vi "Automated5.vi"() -> ()   [LabVIEW 2018]
uses:
  <vilib>/Platform/TimedLoop/XDataNode/timing_clust.ctl
  <vilib>/Platform/TimedLoop/XDataNode/nitl_modes.ctl
  <vilib>/Platform/TimedLoop/XDataNode/wakeup.ctl
  <vilib>/DAQmx/read.llb/DAQmx Read (Analog 1D DBL NChan 1Samp).vi
  <vilib>/DAQmx/create/channels.llb/DAQmx Create Channel (AI-Voltage-Basic).vi
  <vilib>/Enthought/Python Integration Toolkit/api/Unpack Double.vi
  <vilib>/DAQmx/miscellaneous.llb/DAQmx Fill In Error Info.vi
  <vilib>/platform/TimedLoop/XDataNode/XDataNode.xnode
  Program Files/National Instruments/LabVIEW 2015/instr.lib/Omega CN7500/Omega CN7500.lvlib
  <instrlib>/Brooks DLL 64bit/0254 64bit/BrooksDLL64.dll
  <vilib>/Platform/TimedLoop/XDataNode/XDNodeRunTimeDep.lvlib
  <vilib>/Enthought/Python Integration Toolkit/Python Integration Toolkit.lvlib
panel:
  out "CH4/He Set Flow 9":dbl
  out "N2 Set Flow 9":dbl
  out "CH4/He Set Flow 8":dbl
  out "N2 Set Flow 8":dbl
  out "CH4/He Set Flow 7":dbl
  out "N2 Set Flow 7":dbl
  out "CH4/He Set Flow 6":dbl
  out "N2 Set Flow 6":dbl
  out "CH4/He Set Flow 5":dbl
  out "N2 Set Flow 5":dbl
  out "CH4/He Set Flow 4":dbl
  out "N2 Set Flow 4":dbl
  out "CH4/He Set Flow 3":dbl
  out "N2 Set Flow 3":dbl
  out "CH4/He Set Flow 2":dbl
  out "N2 Set Flow 2":dbl
  out "CH4/He Set Flow 1":dbl
  out "N2 Set Flow 1":dbl
  out "CH4/He  Set Flow 0":dbl
  out "N2 Set Flow 0":dbl
  out "New temp":dbl
  out "Previous temp":dbl
  out "Exp 10":bool=TRUE
  in  "CH4/He mole frac 10":dbl
  in  "O2 mole Frac 10":dbl
  out "O2 Flow 10":dbl
  out "CH4/He Actual Flow 10":dbl
  out "N2 mole frac 10":dbl
  out "N2 Actual Flow 10":dbl
  out "Measured CO2 mol fraction 8":dbl
  out "Measured O2 mol fraction 8":dbl
  out "Measured CH4 mol fraction 8":dbl
  out "Exp 9":bool=TRUE
  in  "CH4/He mole frac 9":dbl
  in  "O2 mole Frac 9":dbl
  out "O2 Flow 9":dbl
  out "CH4/He Actual Flow 9":dbl
  out "N2 mole frac 9":dbl
  out "N2 Actual Flow 9":dbl
  out "Temp ShutDown Limit Reached":bool
  out "Pressure ShutDown Limit Reached":bool
  out "Measured CO2 mol fraction 7":dbl
  out "Measured O2 mol fraction 7":dbl
  out "Measured CH4 mol fraction 7":dbl
  out "Exp 8":bool=TRUE
  in  "Temp 8":dbl
  in  "CH4/He mole frac 8":dbl
  in  "Total Flow 8":dbl
  in  "O2 mole Frac 8":dbl
  out "O2 Flow 8":dbl
  out "CH4/He Actual Flow 8":dbl
  out "N2 mole frac 8":dbl
  out "N2 Actual Flow 8":dbl
  out "Measured CO2 mol fraction 6":dbl
  out "Measured O2 mol fraction 6":dbl
  out "Measured CH4 mol fraction 6":dbl
  out "Exp 7":bool=TRUE
  in  "Temp 7":dbl
  in  "CH4/He mole frac 7":dbl
  in  "Total Flow 7":dbl
  in  "O2 mole Frac 7":dbl
  out "O2 Flow 7":dbl
  out "CH4/He Actual Flow 7":dbl
  out "N2 mole frac 7":dbl
  out "N2 Actual Flow 7":dbl
  out "Measured CO2 mol fraction 5":dbl
  out "Measured O2 mol fraction 5":dbl
  out "Measured CH4 mol fraction 5":dbl
  out "Exp 6":bool=TRUE
  in  "Temp 6":dbl
  in  "CH4/He mole frac 6":dbl
  in  "Total Flow 6":dbl
  in  "O2 mole Frac 6":dbl
  out "O2 Flow 6":dbl
  out "CH4/He Actual Flow 6":dbl
  out "N2 mole frac 6":dbl
  out "N2 Actual Flow 6":dbl
  out "Measured CO2 mol fraction 4":dbl
  out "Measured O2 mol fraction 4":dbl
  out "Measured CH4 mol fraction 4":dbl
  out "Exp 5":bool=TRUE
  in  "Temp 5":dbl
  in  "CH4/He mole frac 5":dbl
  in  "Total Flow 5":dbl
  in  "O2 mole Frac 5":dbl
  out "O2 Flow 5":dbl
  out "CH4/He Actual Flow 5":dbl
  out "N2 mole frac 5":dbl
  out "N2 Actual Flow 5":dbl
  out "Measured CO2 mol fraction 3":dbl
  out "Measured O2 mol fraction 3":dbl
  out "Measured CH4 mol fraction 3":dbl
  out "Exp 4":bool=TRUE
  in  "Temp 4":dbl
  in  "CH4/He mole frac 4":dbl
  in  "Total Flow 4":dbl
  in  "O2 mole Frac 4":dbl
  out "O2 Flow 4":dbl
  out "CH4/He Actual Flow 4":dbl
  out "N2 mole frac 4":dbl
  out "N2 Actual Flow 4":dbl
  out "Measured CO2 mol fraction 2":dbl
  out "Measured O2 mol fraction 2":dbl
  out "Measured CH4 mol fraction 2":dbl
  out "Exp 3":bool=TRUE
  in  "Temp 3":dbl
  in  "CH4/He mole frac 3":dbl
  in  "Total Flow 3":dbl
  in  "O2 mole Frac 3":dbl
  out "O2 Flow 3":dbl
  out "CH4/He Actual Flow 3":dbl
  out "N2 mole frac 3":dbl
  out "N2 Actual Flow 3":dbl
  out "Most recent GC number":dbl
  in  "GC Duration (min)":dbl
  out "Measured CH4 mol fraction 1":dbl
  out "Measured O2 mol fraction 1":dbl
  out "Measured CO2 mol fraction 1":dbl
  out "N2 Actual Flow 2":dbl
  out "N2 mole frac 2":dbl
  out "CH4/He Actual Flow 2":dbl
  out "O2 Flow 2":dbl
  in  "O2 mole Frac 2":dbl
  in  "Total Flow 2":dbl
  in  "CH4/He mole frac 2":dbl
  in  "Temp 2":dbl
  out "Exp 2":bool=TRUE
  out "Exp 1":bool=TRUE
  in  "Temp 1":dbl
  in  "CH4/He mole frac 1":dbl
  in  "Total Flow 1":dbl
  in  "O2 mole Frac 1":dbl
  out "O2 Flow 1":dbl
  out "CH4/He Actual Flow 1":dbl
  out "N2 mole frac 1":dbl
  out "N2 Actual Flow 1":dbl
  in  "Catalyst Mass (mg)":sgl
  in  "Result File Name (must include .xlsx)":string
  in  "GC folder file name":string
  out "Pressure safety shut down":dbl=3.0
  in  "Skip Experiment":bool
  out "Shut down Temperature":dbl=400.0
  in  "Shut Down Everything":bool
  in  "Exp Duration (min)":dbl
  in  "SetPoint Ch 1":sgl
  in  "SetPoint Ch2":sgl
  in  "SetPoint Ch3":sgl
  out "N2 Actual Flow 0":dbl
  out "N2 mole frac 0":dbl
  out "CH4/He Actual Flow 0":dbl
  out "O2 Flow 0":dbl
  in  "O2 mole Frac 0":dbl
  in  "Total Flow 0":dbl
  in  "CH4/He mole frac 0":dbl
  in  "Temp 0":dbl
  out "Exp 0":bool=TRUE
  out "Loop Count":i32
  in  "Target Temperaure value":dbl
  in  "Manual or Automatic":bool
  out "Temperature":dynamicdata(graph)
  in  "Update temperature":bool
  out "Temp Process Value":dbl
  out "Inlet Pressure (Bar g) 3":dbl format="%#.3g"
  out "Outlet Pressure (Bar g) 2":dbl format="%#.3g"
  out "Pressure":dynamicdata(graph)
  out "Read SetPoint Ch1":sgl
  out "Process Value Ch1":sgl
  in  "Update Flow set point":bool
  out "Read SetPoint Ch2":sgl
  out "Process Value Ch2":sgl
  out "Read SetPoint Ch3":sgl
  out "Process Value Ch3":sgl
  in  "CN 7500":refnum<visa-resource-name>
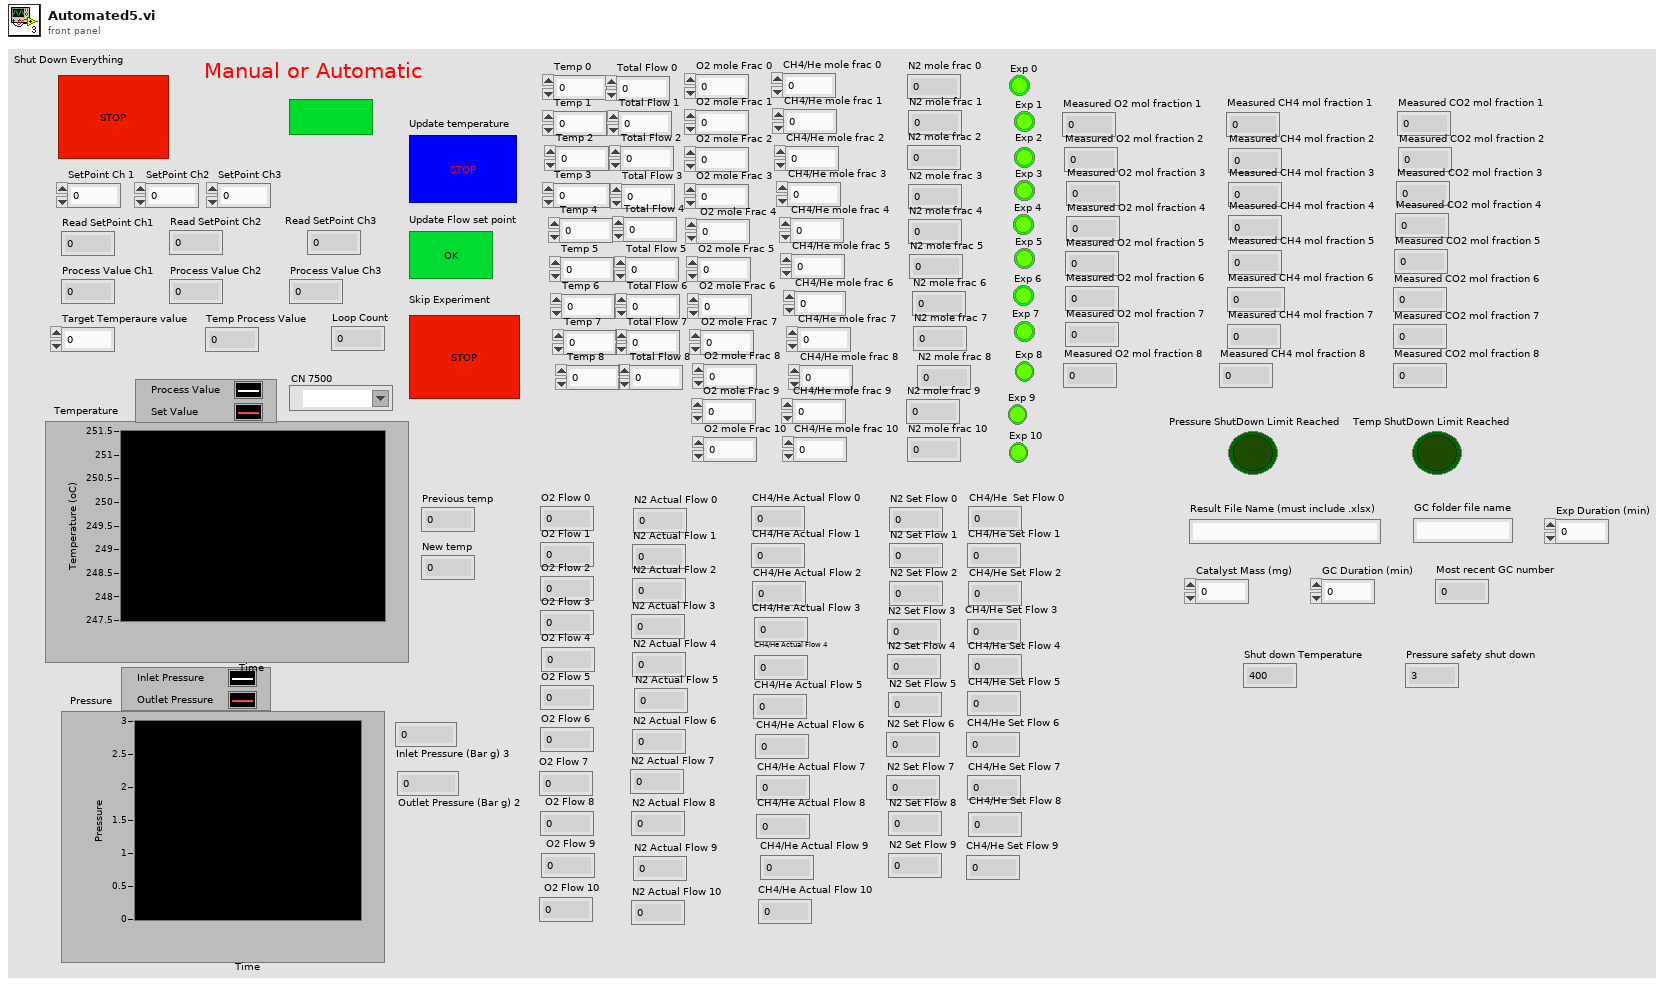
[diagram p1: front panel]
types:
  T1 = typedef "XDNodeRunTimeDep.lvlib/timing_clust.ctl" = cluster{"Expected End [f-1]":u64, "Actual End [f-1]":u64, "Finished Late? [f-1]":bool, "Expected End [i-1]":u64, "Actual End [i-1]":u64, "Finished Late? [i-1]":bool, "Expected Start [i]":u64, "Actual Start [i]":u64, "Expected Start [f]":u64, "Actual Start [f]":u64, "Source Name":string, "Structure Name":string, "Period":i64, "Deadline":i64, "Offset":i64, "Start":i64, "Priority":i32, "Timeout":i32, "Mode":T2, "Wakeup Reason":T3, "Error":errorcluster, "Source Type":string, "Secondary Source Type":string, "Global End Time":u64, "Global Start Time":u64, "Frame Duration":u64, "Iteration Duration":u64, "Assigned CPU":i32, "I/O Scan Engine Mode":u32}
  T2 = typedef "XDNodeRunTimeDep.lvlib/nitl_modes.ctl" = enum32{"No Change", "Process missed periods, maintain original phase", "Discard missed periods, maintain original phase", "Process missed periods, ignore original phase", "Discard missed periods, ignore original phase"}
  T3 = typedef "XDNodeRunTimeDep.lvlib/wakeup.ctl" = enum32{"Normal", "Aborted", "Asynchronous wakeup", "Timing source error", "Timed loop error", "Timeout"}
  T4 = typedef "Python Integration Toolkit.lvlib/Session ID.ctl" = u64
  T5 = typedef "Python Integration Toolkit.lvlib/Python Objects.ctl" = variant
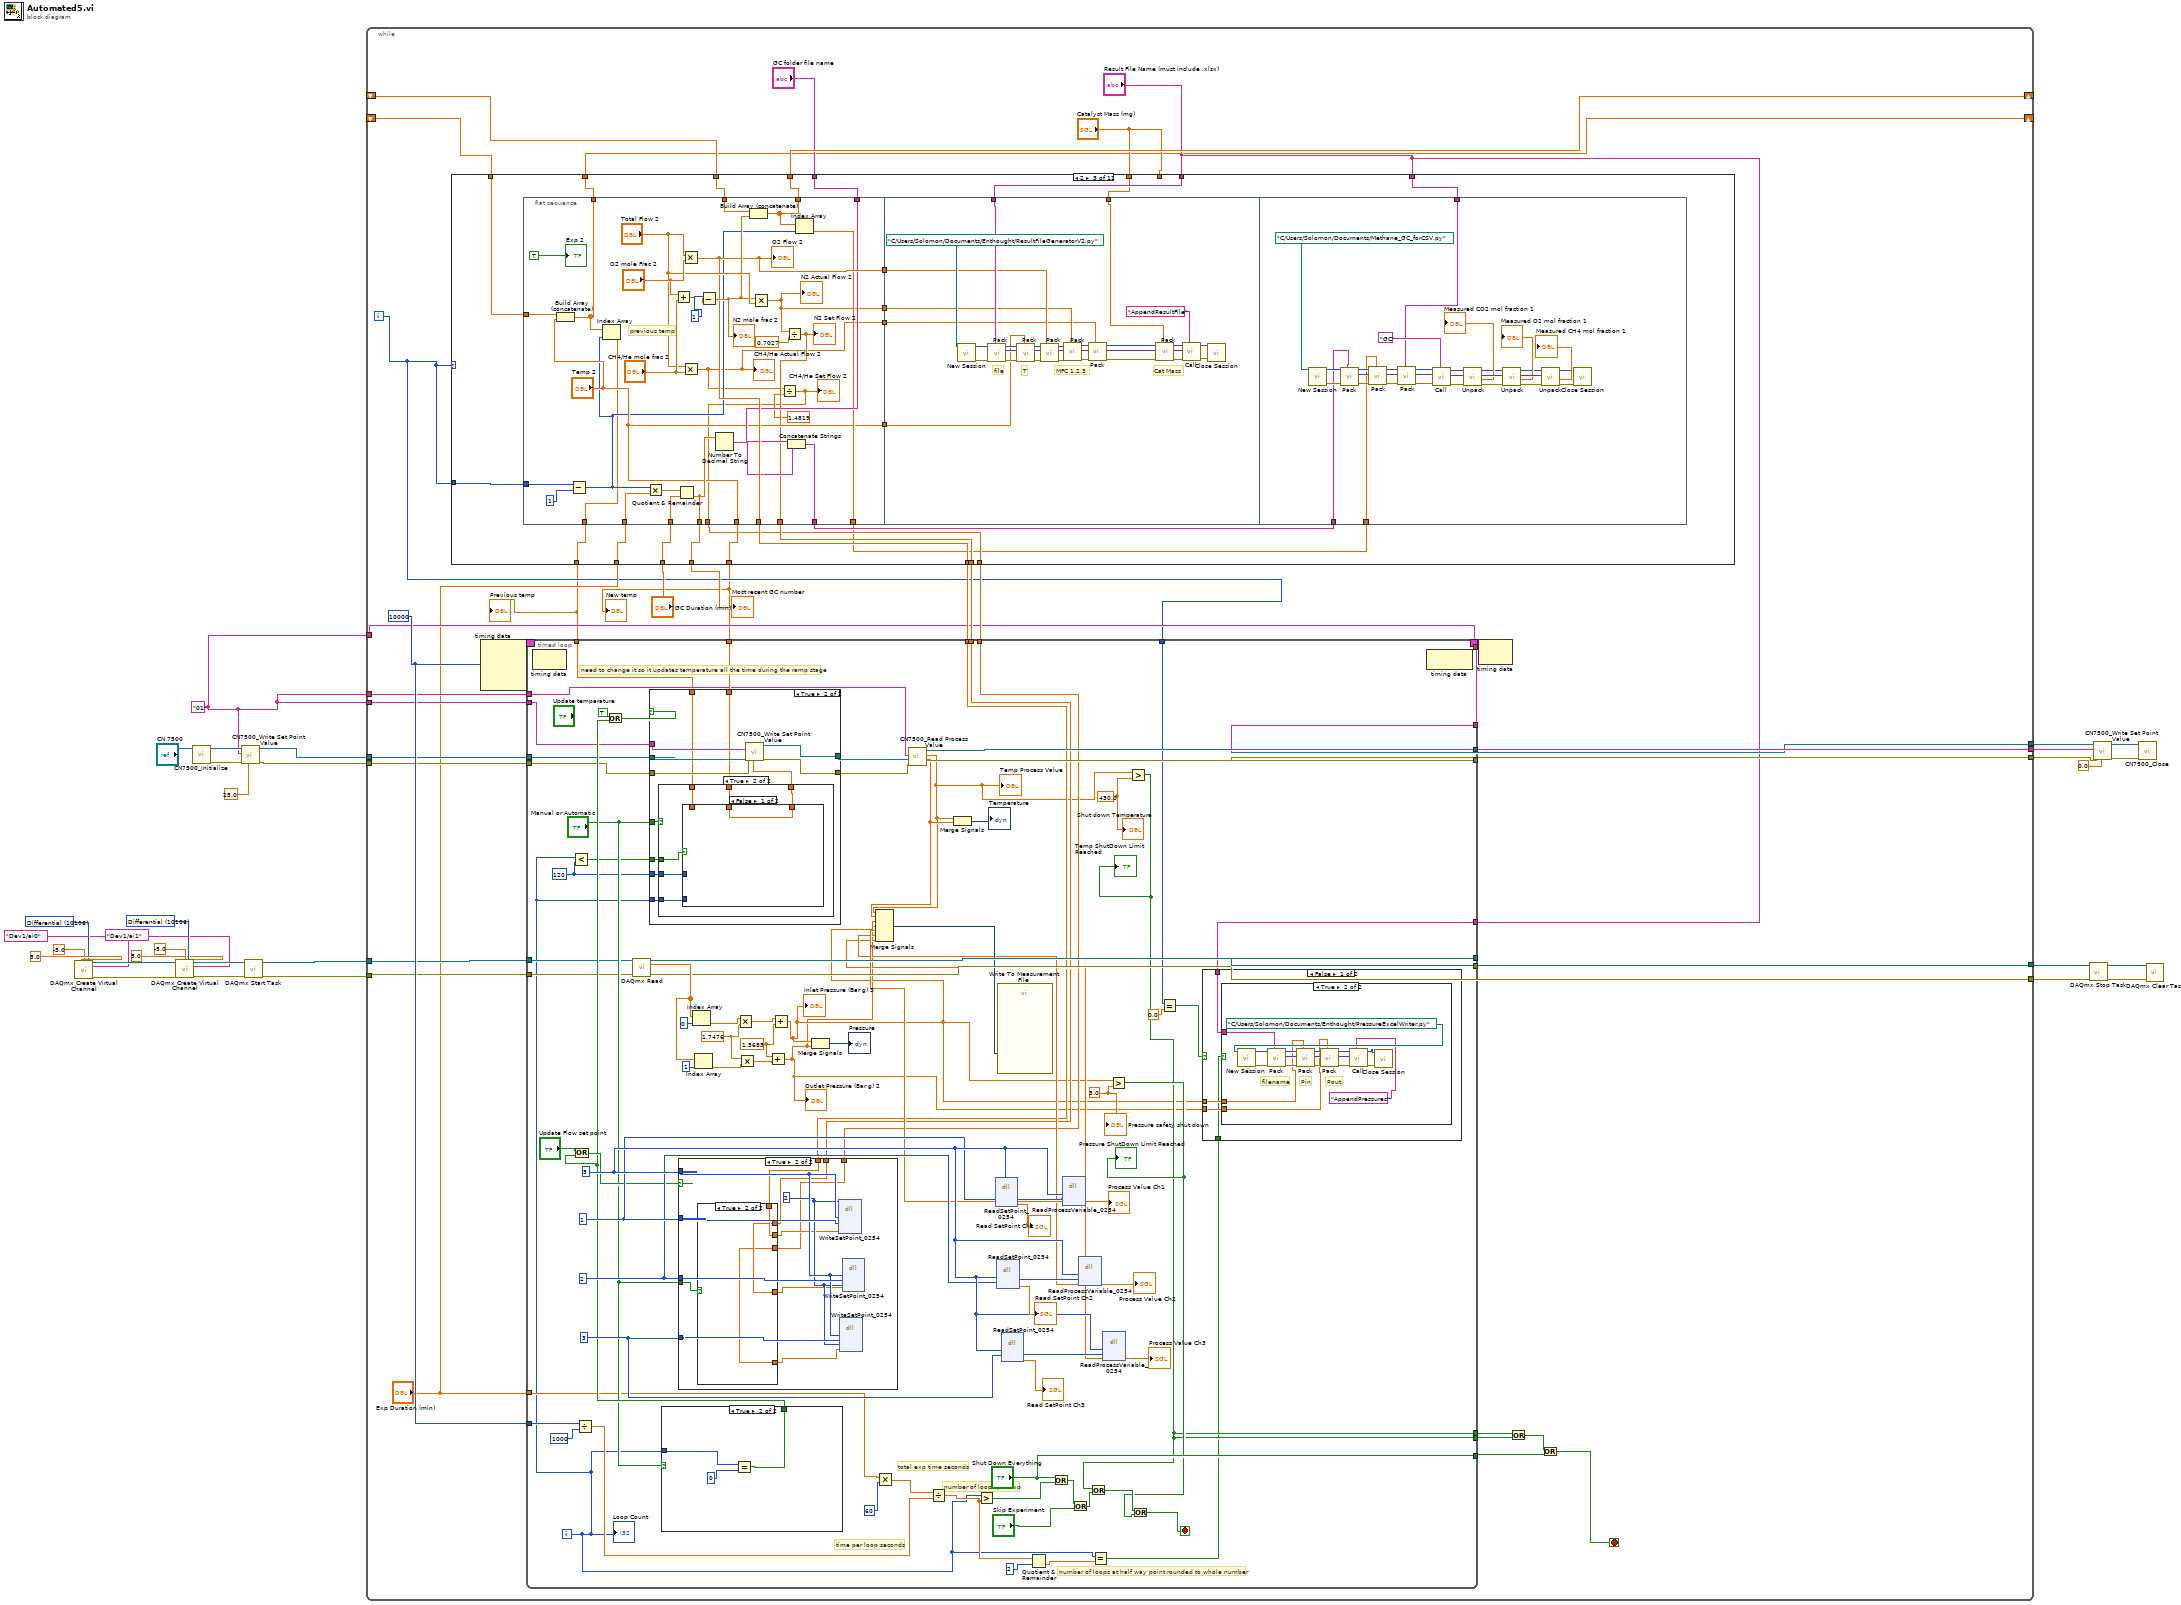
[diagram p0: block diagram]
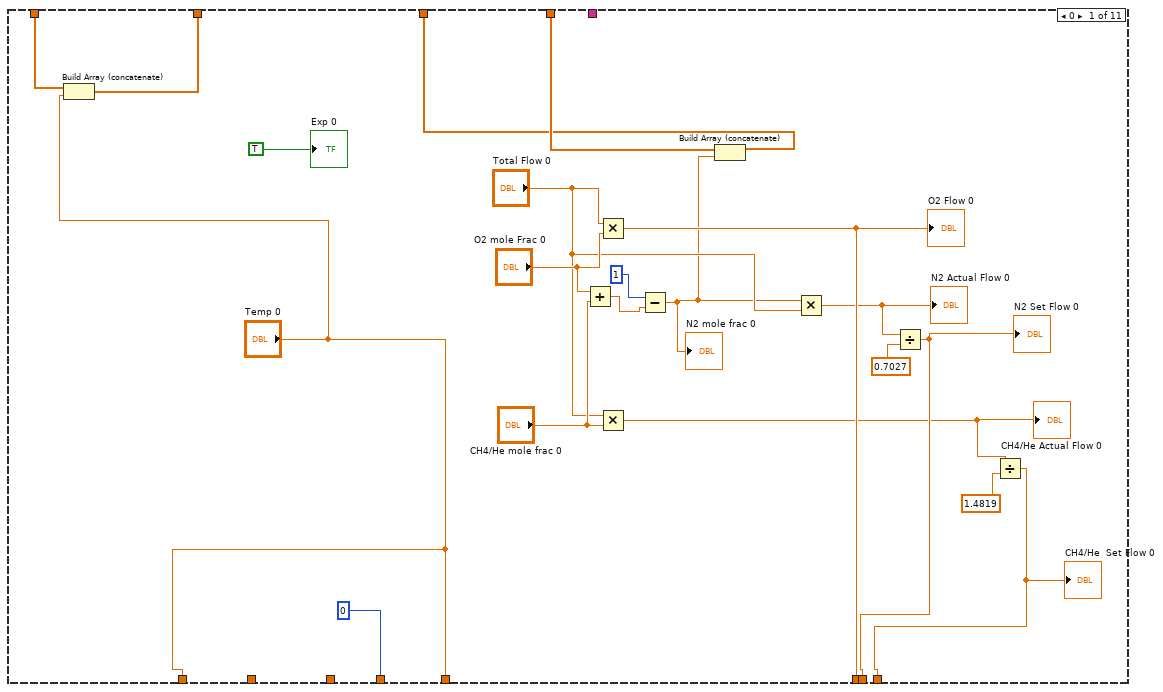
[diagram p2: hidden frame]
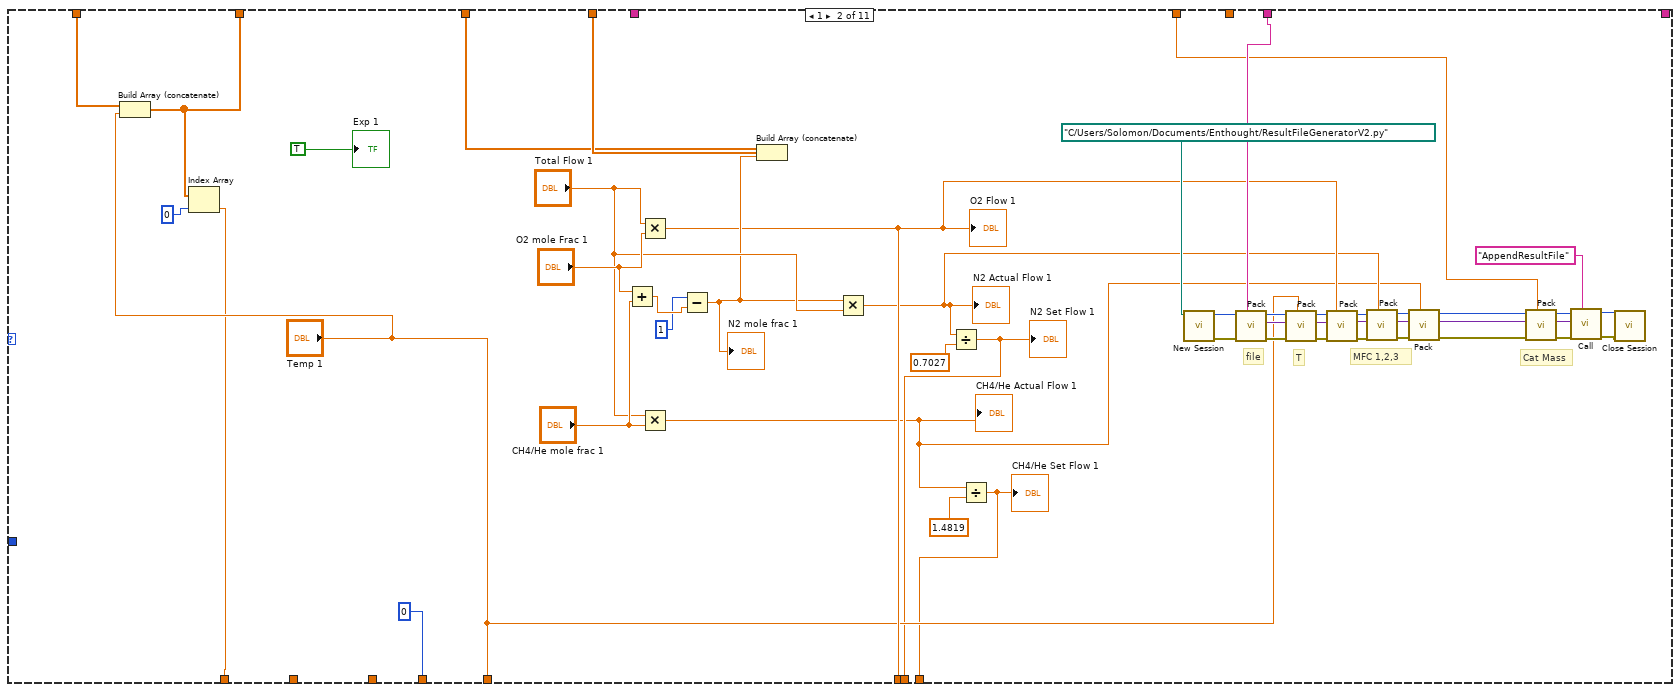
[diagram p3: hidden frame]
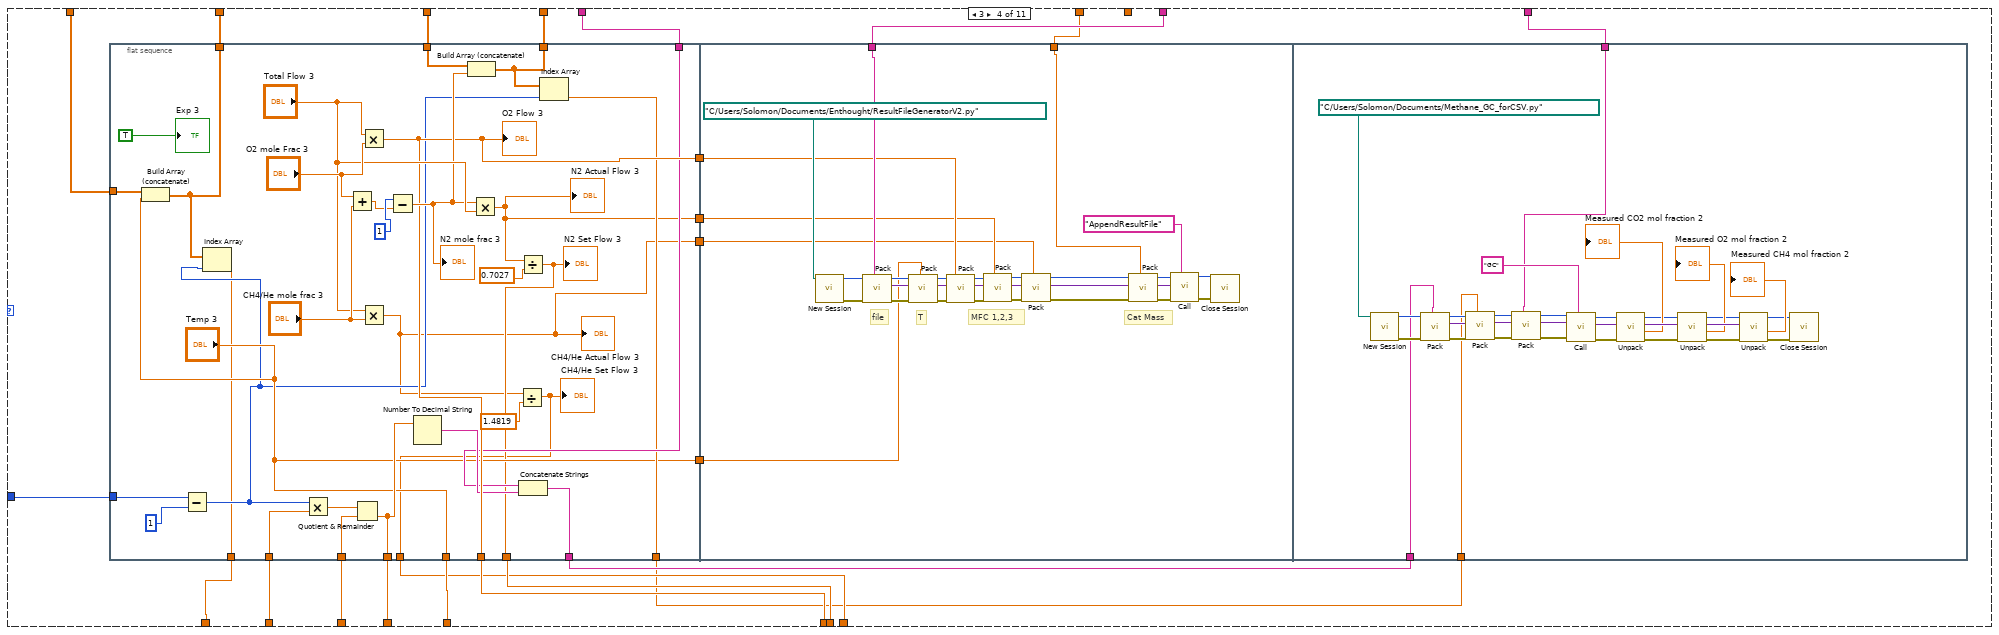
[diagram p4: hidden frame]
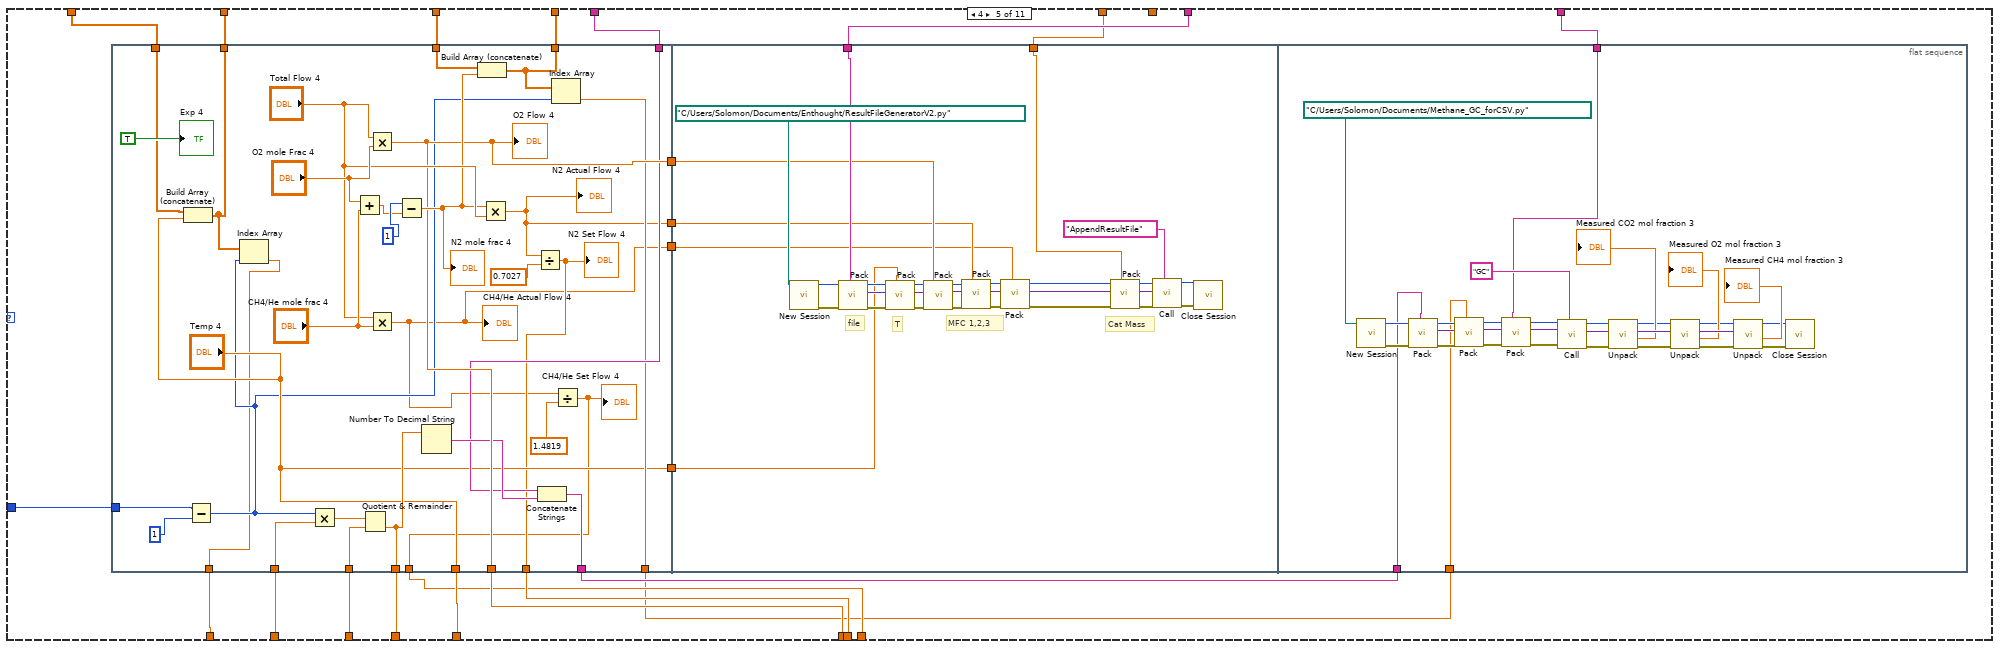
[diagram p5: hidden frame]
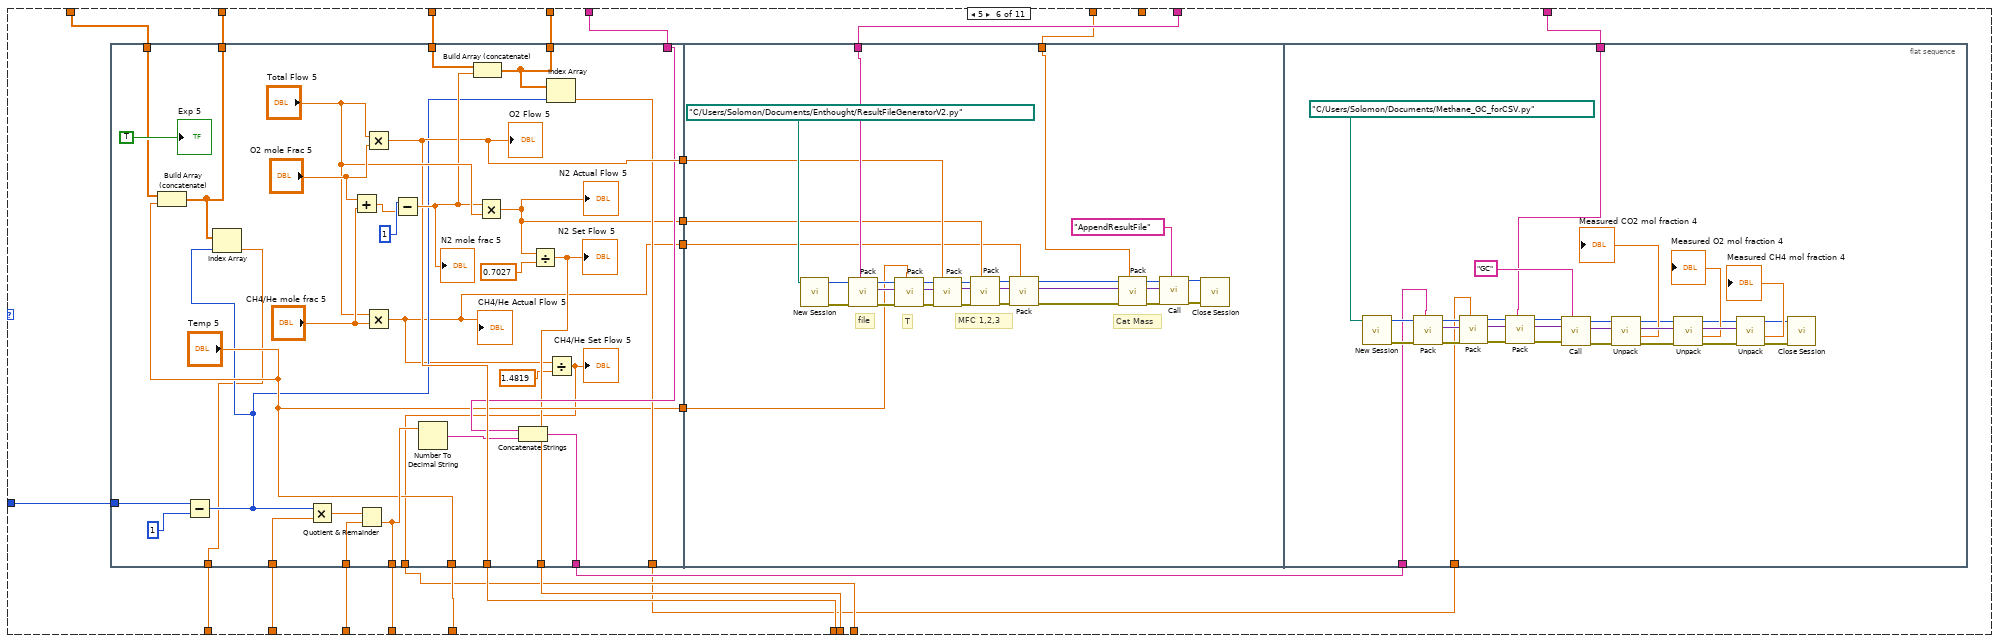
[diagram p6: hidden frame]
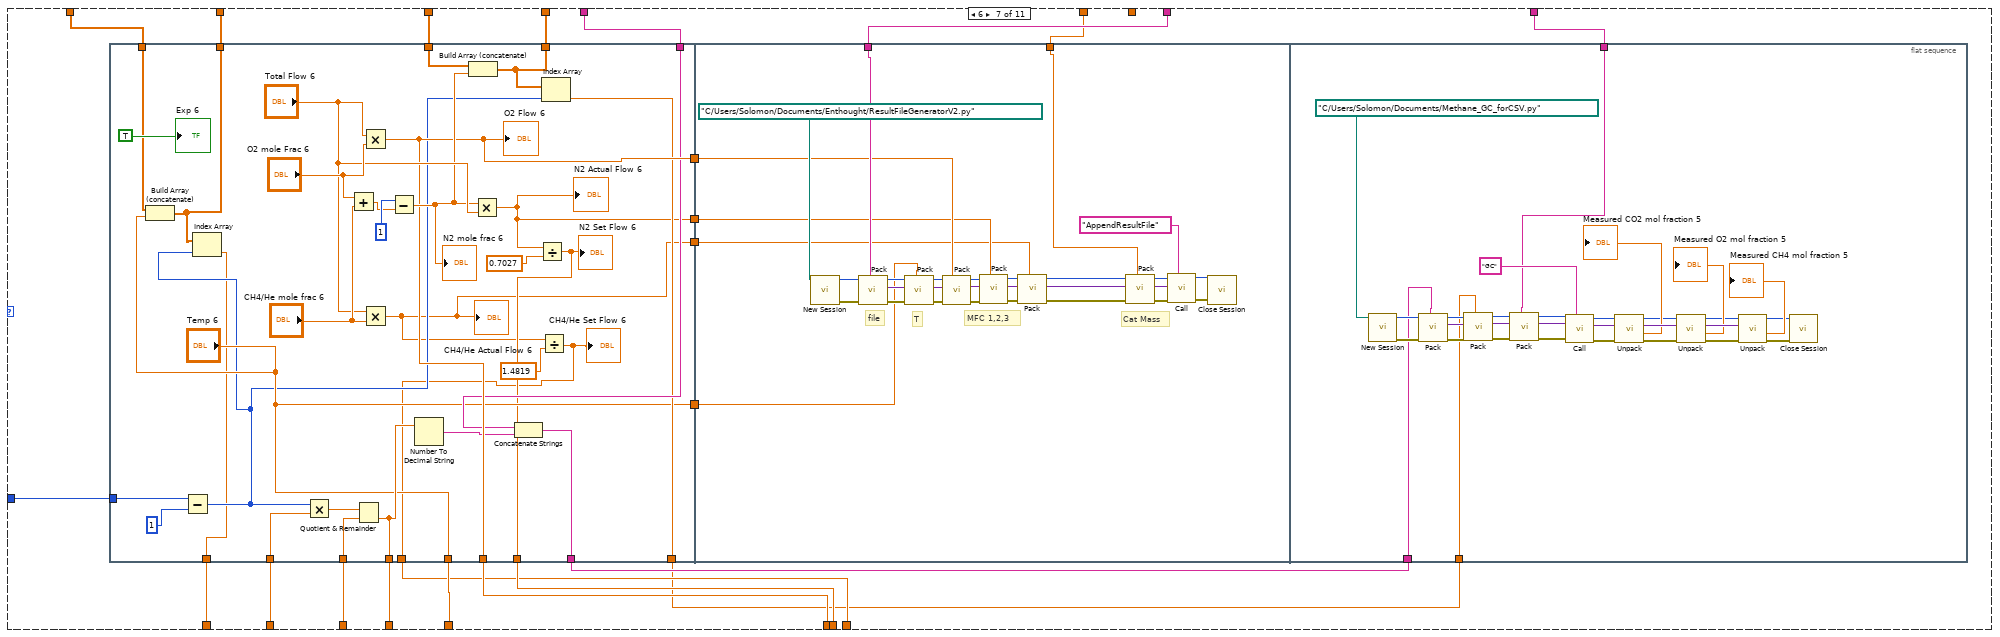
[diagram p7: hidden frame]
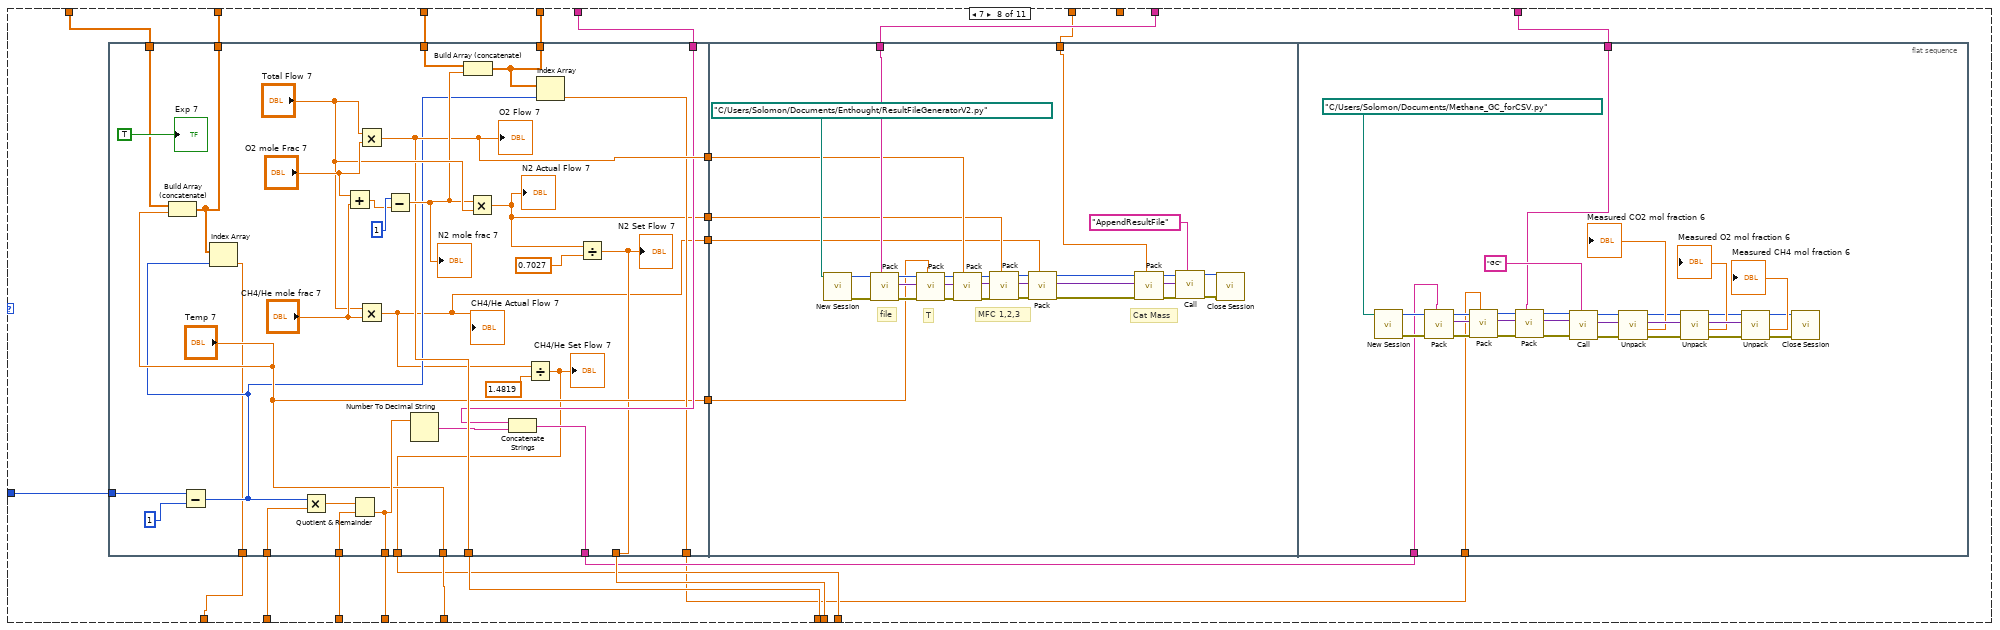
[diagram p8: hidden frame]
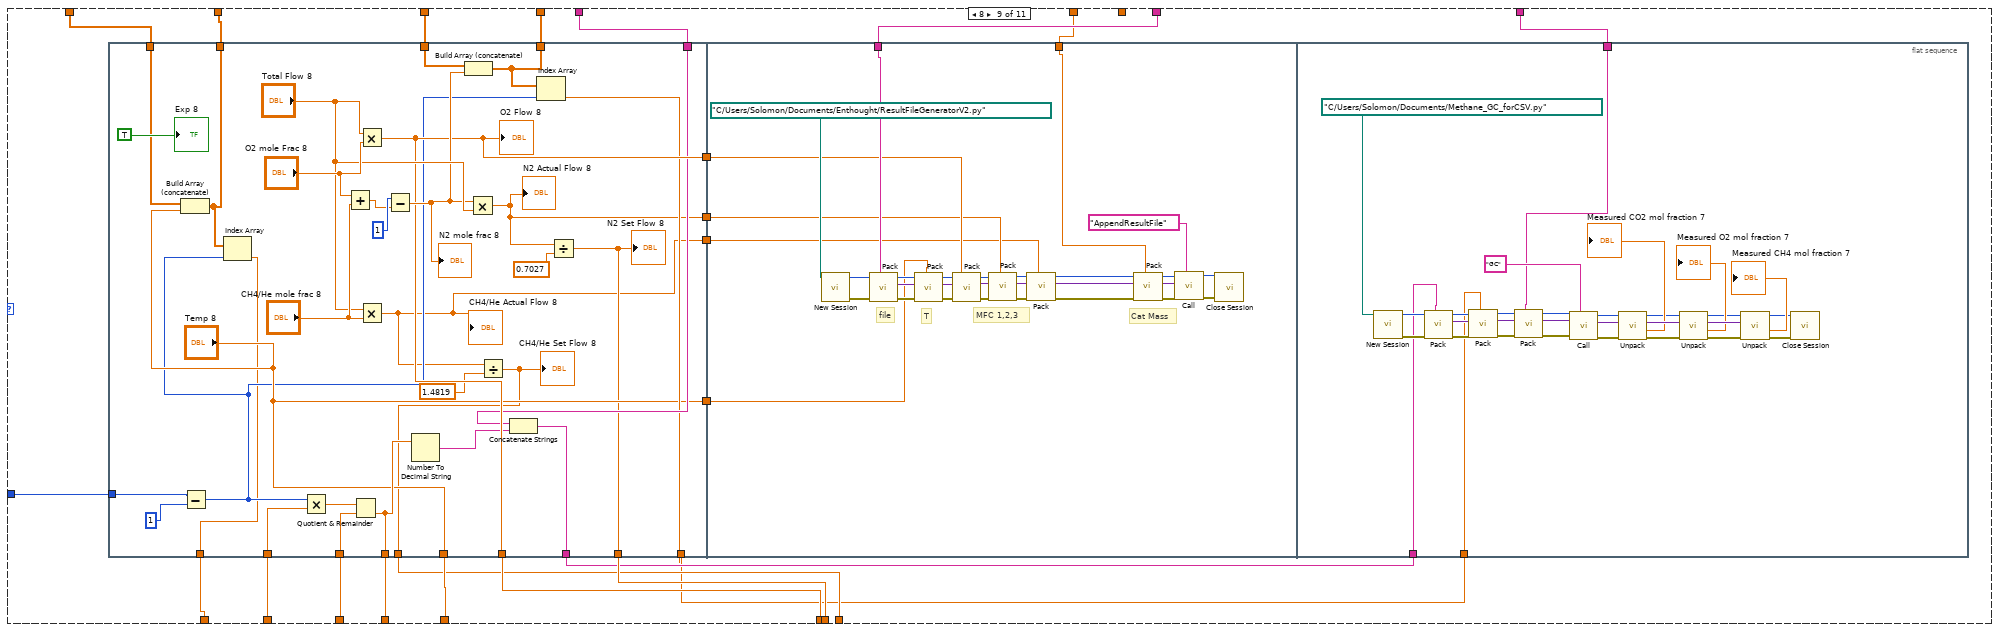
[diagram p9: hidden frame]
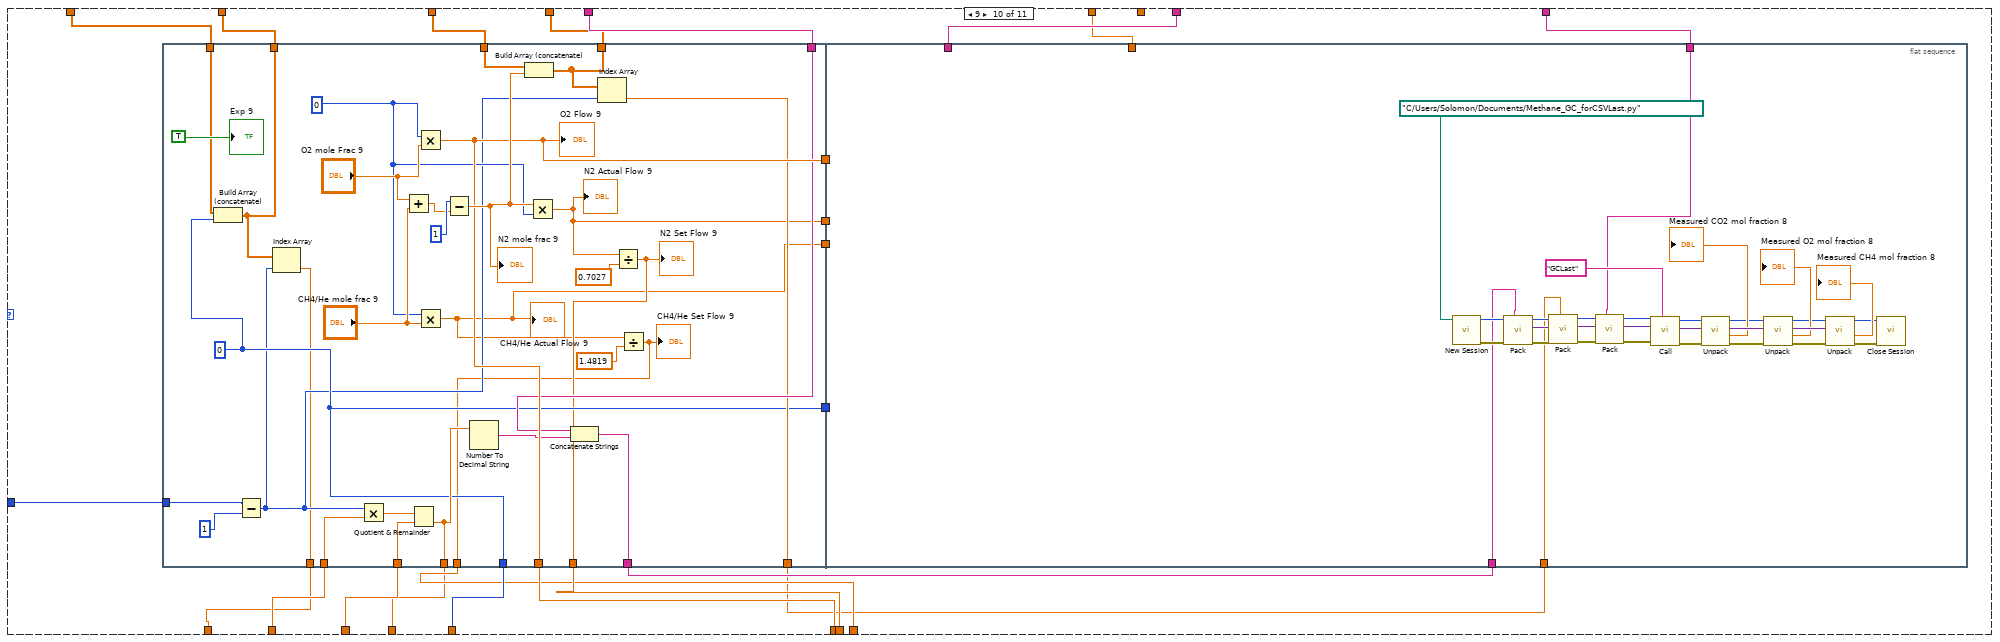
[diagram p10: hidden frame]
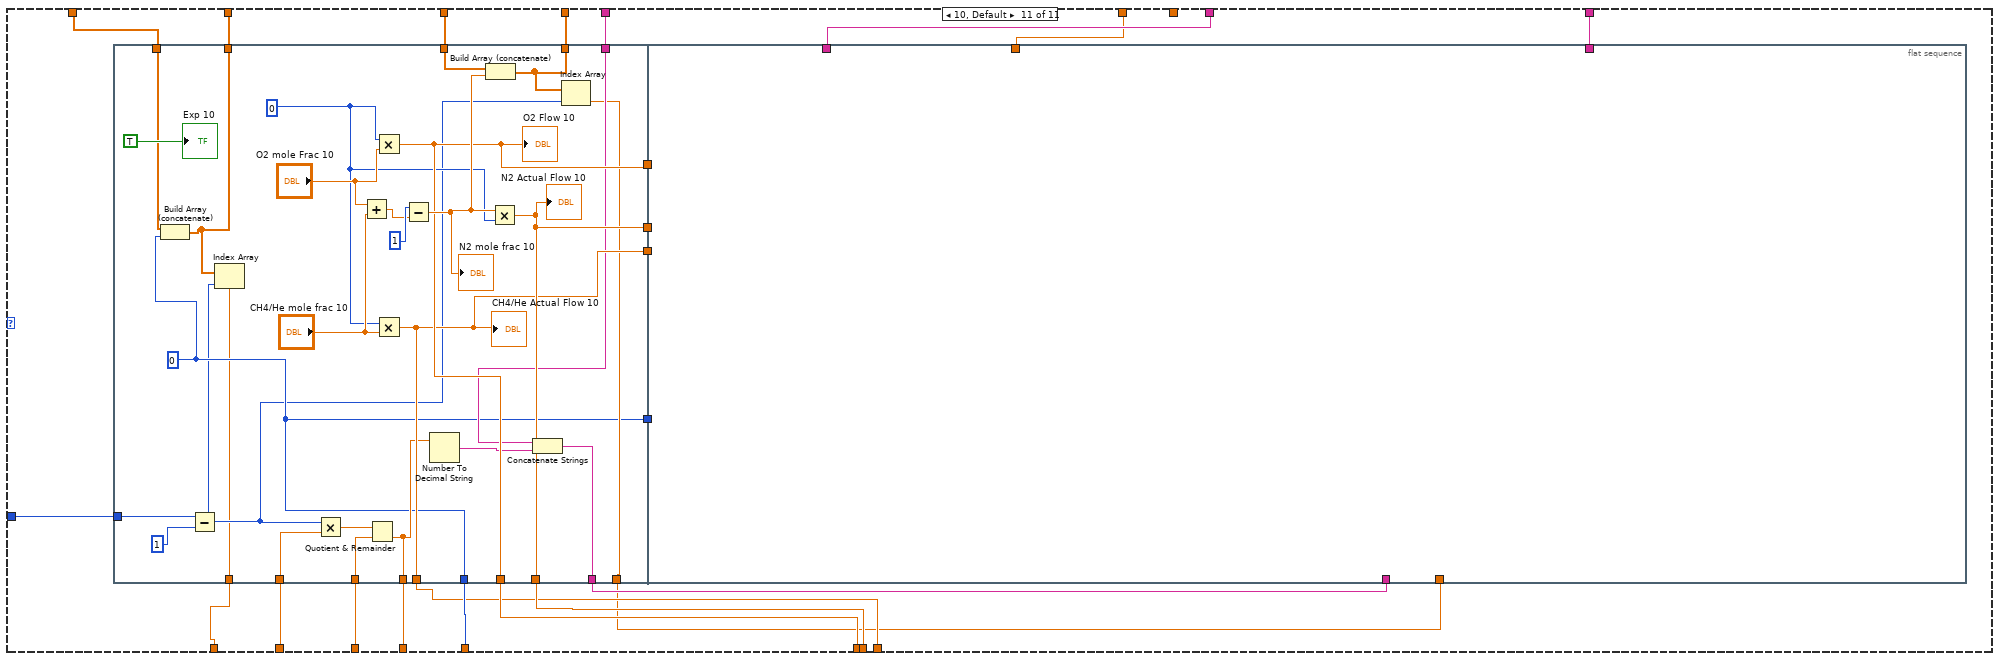
[diagram p11: hidden frame]
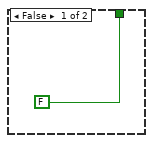
[diagram p14: hidden frame]
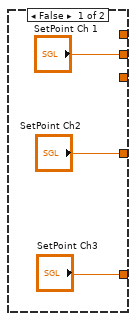
[diagram p16: hidden frame]
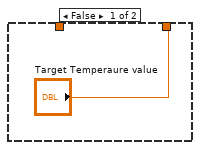
[diagram p18: hidden frame]
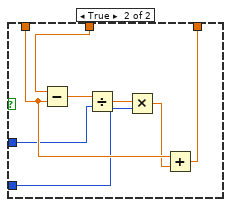
[diagram p19: hidden frame]
diagram:
  w20 = 10106 items=["Default"=-1, "RSE"=10083, "NRSE"=10078, "Differential"=10106, "Pseudodifferential"=12529] ("input terminal configuration")
  w16 = 10106 items=["Default"=-1, "RSE"=10083, "NRSE"=10078, "Differential"=10106, "Pseudodifferential"=12529] ("input terminal configuration")
  w27 = "01" ("Controller Number")
  n1 = call-poly <vilib>:"DAQmx Create Virtual Channel.vi"("maximum value"=5.0, "minimum value"=-5.0, "input terminal configuration"=w16, "physical channels"=tag "Dev1/ai0" ("DAQmx Physical Channel")) -> ("task out"=w22:refnum<k21>, "error out"=w24:errorcluster)  [unwired: 10 in]
  n2 = call-poly <vilib>:"DAQmx Create Virtual Channel.vi"("task in"=w22, "maximum value"=5.0, "minimum value"=-5.0, "input terminal configuration"=w20, "physical channels"=tag "Dev1/ai1" ("DAQmx Physical Channel"), "error in"=w24) -> ("task out"=w23:refnum<k21>, "error out"=w25:errorcluster)  [unwired: 8 in]
  n3 = call "CN7500_Initialize.vi"("VISA resource name"="CN 7500") -> ("error out"=w31:errorcluster, "VISA resource name out"=w30:refnum<visa-resource-name>)  [unwired: 9 in]
  n4 = call "CN7500_Write Set Point Value.vi"("Target Set Point Value"=25.0, "error in (no error)"=w31, "Controller Number"=w27, "VISA In"=w30) -> ("error out"=w26:errorcluster, "VISA Out"=w11:refnum<visa-resource-name>)  [unwired: 6 in]
  n5 = call <vilib>:"DAQmx Start Task.vi"("task/channels in"=w23, "error in"=w25) -> ("task out"=w13:refnum<k21>, "error out"=w14:errorcluster)  [unwired: 12 in]
  n6 = while {
    tunnel: w27 -> [w61]
    tunnel: w27 -> [w60]
    tunnel: w27 -> [w59]
    tunnel: w26 -> [w58]
    tunnel: w14 -> [w57]
    tunnel: w13 -> [w56]
    tunnel: w11 -> [w55]
    shift-right: [w49] -> _
    shift-left: _ -> [w43]
    tunnel: [w42] -> w8
    tunnel: [w41] -> w7
    tunnel: [w40] -> w3
    tunnel: [w39] -> w2
    tunnel: [w38] -> w1
    shift-right: [w34] -> _
    shift-left: _ -> [w35]
    i -> [w36]
    stop <- w50 stop-if-true
    w62 = 10000
    n7 = case shown="2" w36 {
      tunnel: ["Temp 0" "Temp 1" w158 w272 w386 w500 w614 w728 w842 w956 w1040] -> w32
      tunnel: [w83 w106 w156 w270 w384 w498 w612 w726 w840 w954 w1038] -> w65
      tunnel: [w71 w91 w155 w269 w383 w497 w611 w725 w839 w953 w1037] -> w64
      tunnel: [w68 w88 w154 w268 w382 w496 w610 w724 w838 w952 w1036] -> w63
      tunnel: [w81 w130 w141 w255 w369 w483 w597 w711 w825 w939 w1023] -> w49
      tunnel: w43 -> [w80 w129 w157 w271 w385 w499 w613 w727 w841 w955 w1039]
      tunnel: "GC folder file name" -> [_ _ w143 w257 w371 w485 w599 w713 w827 w941 w1025]
      tunnel: "Result File Name (must include .xlsx)" -> [_ w109 w152 w266 w380 w494 w608 w722 w836 w950 w1034]
      tunnel: "Catalyst Mass (mg)" -> [_ _ _ _ _ _ _ _ _ _ _]
      tunnel: "Catalyst Mass (mg)" -> [_ w105 w148 w262 w376 w490 w604 w718 w832 w946 w1030]
      tunnel: w36 -> [_ _ w147 w261 w375 w489 w603 w717 w831 w945 w1029]
      tunnel: "Exp Duration (min)" -> [_ _ w146 w260 w374 w488 w602 w716 w830 w944 w1028]
      tunnel: "GC Duration (min)" -> [_ _ w145 w259 w373 w487 w601 w715 w829 w943 w1027]
      tunnel: [0 0 w144 w258 w372 w486 w600 w714 w828 w942 w1026] -> w44
      tunnel: "Result File Name (must include .xlsx)" -> [_ _ w139 w253 w367 w481 w595 w709 w823 w937 w1021]
      tunnel: w35 -> [w75 w98 w138 w252 w366 w480 w594 w708 w822 w936 w1020]
      tunnel: [w76 w96 w137 w251 w365 w479 w592 w707 w821 w935 w1019] -> w34
      tunnel: ["Temp 0" w94 w136 w250 w364 w478 w593 w706 w820 w934 w1018] -> w33
      frame 0 {
        n8 = Build Array (concatenate)(w75, "Temp 0") -> (w76:dbl[])
        n9 = Add(x="O2 mole Frac 0", y="CH4/He mole frac 0") -> (x+y=w77:dbl)
        n10 = Multiply(x="Total Flow 0", y="O2 mole Frac 0") -> (x*y=w83:dbl)
        "O2 Flow 0" <- w83
        n11 = Multiply(x="Total Flow 0", y="CH4/He mole frac 0") -> (x*y=w70:dbl)
        "CH4/He Actual Flow 0" <- w70
        n12 = Subtract(x=1, y=w77) -> (x-y=w82:dbl)
        "N2 mole frac 0" <- w82
        n13 = Build Array (concatenate)(w80, w82) -> (w81:dbl[])
        n14 = Multiply(x=w82, y="Total Flow 0") -> (x*y=w73:dbl)
        "N2 Actual Flow 0" <- w73
        n15 = Divide(x=w73, y=0.7027) -> (x/y=w71:dbl)
        "N2 Set Flow 0" <- w71
        n16 = Divide(x=w70, y=1.4819) -> (x/y=w68:dbl)
        "CH4/He  Set Flow 0" <- w68
        "Exp 0" <- TRUE
      }
      frame 1 {
        # "Cat Mass"
        # "MFC 1,2,3"
        # "T"
        # "file"
        n17 = Build Array (concatenate)(w98, "Temp 1") -> (w96:dbl[])
        n18 = Index Array(array=w96, index=0) -> (element=w94:dbl)
        n19 = Add(x="O2 mole Frac 1", y="CH4/He mole frac 1") -> (x+y=w103:dbl)
        n20 = Multiply(x="Total Flow 1", y="O2 mole Frac 1") -> (x*y=w106:dbl)
        "O2 Flow 1" <- w106
        n21 = Multiply(x="Total Flow 1", y="CH4/He mole frac 1") -> (x*y=w89:dbl)
        "CH4/He Actual Flow 1" <- w89
        n22 = Subtract(x=1, y=w103) -> (x-y=w131:dbl)
        "N2 mole frac 1" <- w131
        n23 = Build Array (concatenate)(w129, w131) -> (w130:dbl[])
        n24 = Multiply(x=w131, y="Total Flow 1") -> (x*y=w92:dbl)
        "N2 Actual Flow 1" <- w92
        n25 = Divide(x=w92, y=0.7027) -> (x/y=w91:dbl)
        "N2 Set Flow 1" <- w91
        n26 = Divide(x=w89, y=1.4819) -> (x/y=w88:dbl)
        "CH4/He Set Flow 1" <- w88
        n27 = call <vilib>:"New Session.vi"("Path to Python Module (.py File)"=path "C:/Users/Solomon/Documents/Enthought/ResultFileGeneratorV2.py") -> ("error out"=w127:errorcluster, "Session ID out"=w128:T4)  [unwired: 9 in]
        n28 = call <vilib>:"Pack.vi"("Argument"=w109, "error in (no error)"=w127, "Session ID"=w128) -> ("error out"=w125:errorcluster, "Python Object References Out"=w124:T5, "Session ID out"=w126:T4)  [unwired: 6 in]
        n29 = call <vilib>:"Pack.vi"("Argument"="Temp 1", "error in (no error)"=w125, "Python Object References In"=w124, "Session ID"=w126) -> ("error out"=w119:errorcluster, "Python Object References Out"=w120:T5, "Session ID out"=w121:T4)  [unwired: 5 in]
        n30 = call <vilib>:"Pack.vi"("Argument"=w106, "error in (no error)"=w119, "Python Object References In"=w120, "Session ID"=w121) -> ("error out"=w116:errorcluster, "Python Object References Out"=w117:T5, "Session ID out"=w118:T4)  [unwired: 5 in]
        n31 = call <vilib>:"Pack.vi"("Argument"=w92, "error in (no error)"=w116, "Python Object References In"=w117, "Session ID"=w118) -> ("error out"=w113:errorcluster, "Python Object References Out"=w114:T5, "Session ID out"=w115:T4)  [unwired: 5 in]
        n32 = call <vilib>:"Pack.vi"("Argument"=w89, "error in (no error)"=w113, "Python Object References In"=w114, "Session ID"=w115) -> ("error out"=w99:errorcluster, "Python Object References Out"=w100:T5, "Session ID out"=w101:T4)  [unwired: 5 in]
        n33 = call <vilib>:"Pack.vi"("Argument"=w105, "error in (no error)"=w99, "Python Object References In"=w100, "Session ID"=w101) -> ("error out"=w110:errorcluster, "Python Object References Out"=w111:T5, "Session ID out"=w112:T4)  [unwired: 5 in]
        n34 = call <vilib>:"Call.vi"("Function or Method Name"="AppendResultFile" ("Function Name"), "error in (no error)"=w110, "Python Object References In"=w111, "Session ID"=w112) -> ("error out"=w122:errorcluster, "Session ID out"=w123:T4)  [unwired: 5 in, 1 out]
        n35 = call <vilib>:"Close Session.vi"("error in (no error)"=w122, "Session ID"=w123) -> ()  [unwired: 9 in, 1 out]
        "Exp 1" <- TRUE
      }
      frame 2 {
        n36 = flat-sequence {
          tunnel: ["Temp 2"] -> w158
          tunnel: w157 -> [w184]
          tunnel: [w183] -> w156
          tunnel: [w162] -> w155
          tunnel: [w159] -> w154
          tunnel: ["Temp 2"] -> w153
          tunnel: [w183] -> w151
          tunnel: [w163] -> w150
          tunnel: [w160] -> w149
          tunnel: w147 -> [w182]
          tunnel: w146 -> [w180]
          tunnel: w145 -> [w178]
          tunnel: [w177] -> w144
          tunnel: w143 -> [w175]
          tunnel: [w174] -> w142
          tunnel: [w173] -> w141
          tunnel: [w172] -> w140
          tunnel: w138 -> [w168]
          tunnel: [w167] -> w137
          tunnel: [w165] -> w136
          tunnel: w153 -> [w199]
          tunnel: w152 -> [w197]
          tunnel: w151 -> [w196]
          tunnel: w150 -> [w195]
          tunnel: w149 -> [w194]
          tunnel: w148 -> [w193]
          tunnel: w142 -> [w222]
          tunnel: w140 -> [w221]
          tunnel: w139 -> [w220]
          frame #0 {
            # "previous temp"
            n37 = Build Array (concatenate)(w168, "Temp 2") -> (w167:dbl[])
            n38 = Subtract(x=w182, y=1) -> (x-y=w166:i32)
            n39 = Index Array(array=w167, index=w166) -> (element=w165:dbl)
            n40 = Multiply(x=w166, y=w180) -> (x*y=w179:dbl)
            n41 = Add(x="O2 mole Frac 2", y="CH4/He mole frac 2") -> (x+y=w170:dbl)
            n42 = Quotient & Remainder(x=w179, y=w178) -> (floor(x/y)=w177:dbl)  [unwired: 1 out]
            n43 = Multiply(x="Total Flow 2", y="O2 mole Frac 2") -> (x*y=w183:dbl)
            "O2 Flow 2" <- w183
            n44 = Multiply(x="Total Flow 2", y="CH4/He mole frac 2") -> (x*y=w160:dbl)
            "CH4/He Actual Flow 2" <- w160
            n45 = Subtract(x=1, y=w170) -> (x-y=w185:dbl)
            "N2 mole frac 2" <- w185
            n46 = Number To Decimal String(number=w177) -> (decimal integer string=w176:string)  [unwired: 1 in]
            n47 = Build Array (concatenate)(w184, w185) -> (w173:dbl[])
            n48 = Multiply(x=w185, y="Total Flow 2") -> (x*y=w163:dbl)
            "N2 Actual Flow 2" <- w163
            n49 = Divide(x=w160, y=1.4819) -> (x/y=w159:dbl)
            "CH4/He Set Flow 2" <- w159
            n50 = Divide(x=w163, y=0.7027) -> (x/y=w162:dbl)
            "N2 Set Flow 2" <- w162
            n51 = Concatenate Strings(w175, w176) -> (w174:string)
            n52 = Index Array(array=w173, index=w166) -> (element=w172:dbl)
            "Exp 2" <- TRUE
          }
          frame #1 {
            # "Cat Mass"
            # "MFC 1,2,3"
            # "T"
            # "file"
            n53 = call <vilib>:"New Session.vi"("Path to Python Module (.py File)"=path "C:/Users/Solomon/Documents/Enthought/ResultFileGeneratorV2.py") -> ("error out"=w218:errorcluster, "Session ID out"=w219:T4)  [unwired: 9 in]
            n54 = call <vilib>:"Pack.vi"("Argument"=w197, "error in (no error)"=w218, "Session ID"=w219) -> ("error out"=w216:errorcluster, "Python Object References Out"=w215:T5, "Session ID out"=w217:T4)  [unwired: 6 in]
            n55 = call <vilib>:"Pack.vi"("Argument"=w199, "error in (no error)"=w216, "Python Object References In"=w215, "Session ID"=w217) -> ("error out"=w210:errorcluster, "Python Object References Out"=w211:T5, "Session ID out"=w212:T4)  [unwired: 5 in]
            n56 = call <vilib>:"Pack.vi"("Argument"=w196, "error in (no error)"=w210, "Python Object References In"=w211, "Session ID"=w212) -> ("error out"=w207:errorcluster, "Python Object References Out"=w208:T5, "Session ID out"=w209:T4)  [unwired: 5 in]
            n57 = call <vilib>:"Pack.vi"("Argument"=w195, "error in (no error)"=w207, "Python Object References In"=w208, "Session ID"=w209) -> ("error out"=w204:errorcluster, "Python Object References Out"=w205:T5, "Session ID out"=w206:T4)  [unwired: 5 in]
            n58 = call <vilib>:"Pack.vi"("Argument"=w194, "error in (no error)"=w204, "Python Object References In"=w205, "Session ID"=w206) -> ("error out"=w190:errorcluster, "Python Object References Out"=w191:T5, "Session ID out"=w192:T4)  [unwired: 5 in]
            n59 = call <vilib>:"Pack.vi"("Argument"=w193, "error in (no error)"=w190, "Python Object References In"=w191, "Session ID"=w192) -> ("error out"=w201:errorcluster, "Python Object References Out"=w202:T5, "Session ID out"=w203:T4)  [unwired: 5 in]
            n60 = call <vilib>:"Call.vi"("Function or Method Name"="AppendResultFile" ("Function Name"), "error in (no error)"=w201, "Python Object References In"=w202, "Session ID"=w203) -> ("error out"=w213:errorcluster, "Session ID out"=w214:T4)  [unwired: 5 in, 1 out]
            n61 = call <vilib>:"Close Session.vi"("error in (no error)"=w213, "Session ID"=w214) -> ()  [unwired: 9 in, 1 out]
          }
          frame #2 {
            n62 = call <vilib>:"New Session.vi"("Path to Python Module (.py File)"=path "C:/Users/Solomon/Documents/Methane_GC_forCSV.py") -> ("error out"=w233:errorcluster, "Session ID out"=w231:T4)  [unwired: 9 in]
            n63 = call <vilib>:"Pack.vi"("Argument"=w222, "error in (no error)"=w233, "Session ID"=w231) -> ("error out"=w236:errorcluster, "Python Object References Out"=w246:T5, "Session ID out"=w235:T4)  [unwired: 6 in]
            n64 = call <vilib>:"Pack.vi"("Argument"=w221, "error in (no error)"=w236, "Python Object References In"=w246, "Session ID"=w235) -> ("error out"=w227:errorcluster, "Python Object References Out"=w228:T5, "Session ID out"=w229:T4)  [unwired: 5 in]
            n65 = call <vilib>:"Pack.vi"("Argument"=w220, "error in (no error)"=w227, "Python Object References In"=w228, "Session ID"=w229) -> ("error out"=w226:errorcluster, "Python Object References Out"=w225:T5, "Session ID out"=w224:T4)  [unwired: 5 in]
            n66 = call <vilib>:"Call.vi"("Function or Method Name"="GC" ("Function Name"), "error in (no error)"=w226, "Python Object References In"=w225, "Session ID"=w224) -> ("error out"=w240:errorcluster, "Python Object References Out"=w247:T5, "Session ID out"=w237:T4)  [unwired: 5 in]
            n67 = call-poly <vilib>:"Unpack.vi"("error in (no error)"=w240, "Python Object References In"=w247, "Session ID"=w237) -> ("error out"=w241:errorcluster, "Value"=→"Measured CO2 mol fraction 1":dbl, "Python Object References Out"=w248:T5, "Session ID out"=w238:T4)  [unwired: 5 in]
            n68 = call-poly <vilib>:"Unpack.vi"("error in (no error)"=w241, "Python Object References In"=w248, "Session ID"=w238) -> ("error out"=w242:errorcluster, "Value"=→"Measured O2 mol fraction 1":dbl, "Python Object References Out"=w249:T5, "Session ID out"=w239:T4)  [unwired: 5 in]
            n69 = call-poly <vilib>:"Unpack.vi"("error in (no error)"=w242, "Python Object References In"=w249, "Session ID"=w239) -> ("error out"=w234:errorcluster, "Value"=→"Measured CH4 mol fraction 1":dbl, "Session ID out"=w232:T4)  [unwired: 5 in, 1 out]
            n70 = call <vilib>:"Close Session.vi"("error in (no error)"=w234, "Session ID"=w232) -> ()  [unwired: 9 in, 1 out]
          }
        }
      }
      frame 3 {
        n71 = flat-sequence {
          tunnel: ["Temp 3"] -> w272
          tunnel: w271 -> [w298]
          tunnel: [w297] -> w270
          tunnel: [w276] -> w269
          tunnel: [w273] -> w268
          tunnel: ["Temp 3"] -> w267
          tunnel: [w297] -> w265
          tunnel: [w277] -> w264
          tunnel: [w274] -> w263
          tunnel: w261 -> [w296]
          tunnel: w260 -> [w294]
          tunnel: w259 -> [w292]
          tunnel: [w291] -> w258
          tunnel: w257 -> [w289]
          tunnel: [w288] -> w256
          tunnel: [w287] -> w255
          tunnel: [w286] -> w254
          tunnel: w252 -> [w283]
          tunnel: [w281] -> w251
          tunnel: [w279] -> w250
          tunnel: w267 -> [w313]
          tunnel: w266 -> [w311]
          tunnel: w265 -> [w310]
          tunnel: w264 -> [w309]
          tunnel: w263 -> [w308]
          tunnel: w262 -> [w307]
          tunnel: w256 -> [w336]
          tunnel: w254 -> [w335]
          tunnel: w253 -> [w334]
          frame #0 {
            n72 = Build Array (concatenate)(w283, "Temp 3") -> (w281:dbl[])
            n73 = Subtract(x=w296, y=1) -> (x-y=w280:i32)
            n74 = Index Array(array=w281, index=w280) -> (element=w279:dbl)
            n75 = Multiply(x=w280, y=w294) -> (x*y=w293:dbl)
            n76 = Add(x="O2 mole Frac 3", y="CH4/He mole frac 3") -> (x+y=w284:dbl)
            n77 = Quotient & Remainder(x=w293, y=w292) -> (floor(x/y)=w291:dbl)  [unwired: 1 out]
            n78 = Multiply(x="Total Flow 3", y="O2 mole Frac 3") -> (x*y=w297:dbl)
            "O2 Flow 3" <- w297
            n79 = Multiply(x="Total Flow 3", y="CH4/He mole frac 3") -> (x*y=w274:dbl)
            "CH4/He Actual Flow 3" <- w274
            n80 = Subtract(x=1, y=w284) -> (x-y=w299:dbl)
            "N2 mole frac 3" <- w299
            n81 = Number To Decimal String(number=w291) -> (decimal integer string=w290:string)  [unwired: 1 in]
            n82 = Build Array (concatenate)(w298, w299) -> (w287:dbl[])
            n83 = Multiply(x=w299, y="Total Flow 3") -> (x*y=w277:dbl)
            "N2 Actual Flow 3" <- w277
            n84 = Divide(x=w274, y=1.4819) -> (x/y=w273:dbl)
            "CH4/He Set Flow 3" <- w273
            n85 = Divide(x=w277, y=0.7027) -> (x/y=w276:dbl)
            "N2 Set Flow 3" <- w276
            n86 = Concatenate Strings(w289, w290) -> (w288:string)
            n87 = Index Array(array=w287, index=w280) -> (element=w286:dbl)
            "Exp 3" <- TRUE
          }
          frame #1 {
            # "Cat Mass"
            # "MFC 1,2,3"
            # "T"
            # "file"
            n88 = call <vilib>:"New Session.vi"("Path to Python Module (.py File)"=path "C:/Users/Solomon/Documents/Enthought/ResultFileGeneratorV2.py") -> ("error out"=w332:errorcluster, "Session ID out"=w333:T4)  [unwired: 9 in]
            n89 = call <vilib>:"Pack.vi"("Argument"=w311, "error in (no error)"=w332, "Session ID"=w333) -> ("error out"=w330:errorcluster, "Python Object References Out"=w329:T5, "Session ID out"=w331:T4)  [unwired: 6 in]
            n90 = call <vilib>:"Pack.vi"("Argument"=w313, "error in (no error)"=w330, "Python Object References In"=w329, "Session ID"=w331) -> ("error out"=w324:errorcluster, "Python Object References Out"=w325:T5, "Session ID out"=w326:T4)  [unwired: 5 in]
            n91 = call <vilib>:"Pack.vi"("Argument"=w310, "error in (no error)"=w324, "Python Object References In"=w325, "Session ID"=w326) -> ("error out"=w321:errorcluster, "Python Object References Out"=w322:T5, "Session ID out"=w323:T4)  [unwired: 5 in]
            n92 = call <vilib>:"Pack.vi"("Argument"=w309, "error in (no error)"=w321, "Python Object References In"=w322, "Session ID"=w323) -> ("error out"=w318:errorcluster, "Python Object References Out"=w319:T5, "Session ID out"=w320:T4)  [unwired: 5 in]
            n93 = call <vilib>:"Pack.vi"("Argument"=w308, "error in (no error)"=w318, "Python Object References In"=w319, "Session ID"=w320) -> ("error out"=w304:errorcluster, "Python Object References Out"=w305:T5, "Session ID out"=w306:T4)  [unwired: 5 in]
            n94 = call <vilib>:"Pack.vi"("Argument"=w307, "error in (no error)"=w304, "Python Object References In"=w305, "Session ID"=w306) -> ("error out"=w315:errorcluster, "Python Object References Out"=w316:T5, "Session ID out"=w317:T4)  [unwired: 5 in]
            n95 = call <vilib>:"Call.vi"("Function or Method Name"="AppendResultFile" ("Function Name"), "error in (no error)"=w315, "Python Object References In"=w316, "Session ID"=w317) -> ("error out"=w327:errorcluster, "Session ID out"=w328:T4)  [unwired: 5 in, 1 out]
            n96 = call <vilib>:"Close Session.vi"("error in (no error)"=w327, "Session ID"=w328) -> ()  [unwired: 9 in, 1 out]
          }
          frame #2 {
            n97 = call <vilib>:"New Session.vi"("Path to Python Module (.py File)"=path "C:/Users/Solomon/Documents/Methane_GC_forCSV.py") -> ("error out"=w347:errorcluster, "Session ID out"=w345:T4)  [unwired: 9 in]
            n98 = call <vilib>:"Pack.vi"("Argument"=w336, "error in (no error)"=w347, "Session ID"=w345) -> ("error out"=w350:errorcluster, "Python Object References Out"=w360:T5, "Session ID out"=w349:T4)  [unwired: 6 in]
            n99 = call <vilib>:"Pack.vi"("Argument"=w335, "error in (no error)"=w350, "Python Object References In"=w360, "Session ID"=w349) -> ("error out"=w341:errorcluster, "Python Object References Out"=w342:T5, "Session ID out"=w343:T4)  [unwired: 5 in]
            n100 = call <vilib>:"Pack.vi"("Argument"=w334, "error in (no error)"=w341, "Python Object References In"=w342, "Session ID"=w343) -> ("error out"=w340:errorcluster, "Python Object References Out"=w339:T5, "Session ID out"=w338:T4)  [unwired: 5 in]
            n101 = call <vilib>:"Call.vi"("Function or Method Name"="GC" ("Function Name"), "error in (no error)"=w340, "Python Object References In"=w339, "Session ID"=w338) -> ("error out"=w354:errorcluster, "Python Object References Out"=w361:T5, "Session ID out"=w351:T4)  [unwired: 5 in]
            n102 = call-poly <vilib>:"Unpack.vi"("error in (no error)"=w354, "Python Object References In"=w361, "Session ID"=w351) -> ("error out"=w355:errorcluster, "Value"=→"Measured CO2 mol fraction 2":dbl, "Python Object References Out"=w362:T5, "Session ID out"=w352:T4)  [unwired: 5 in]
            n103 = call-poly <vilib>:"Unpack.vi"("error in (no error)"=w355, "Python Object References In"=w362, "Session ID"=w352) -> ("error out"=w356:errorcluster, "Value"=→"Measured O2 mol fraction 2":dbl, "Python Object References Out"=w363:T5, "Session ID out"=w353:T4)  [unwired: 5 in]
            n104 = call-poly <vilib>:"Unpack.vi"("error in (no error)"=w356, "Python Object References In"=w363, "Session ID"=w353) -> ("error out"=w348:errorcluster, "Value"=→"Measured CH4 mol fraction 2":dbl, "Session ID out"=w346:T4)  [unwired: 5 in, 1 out]
            n105 = call <vilib>:"Close Session.vi"("error in (no error)"=w348, "Session ID"=w346) -> ()  [unwired: 9 in, 1 out]
          }
        }
      }
      frame 4 {
        n106 = flat-sequence {
          tunnel: ["Temp 4"] -> w386
          tunnel: w385 -> [w412]
          tunnel: [w411] -> w384
          tunnel: [w390] -> w383
          tunnel: [w387] -> w382
          tunnel: ["Temp 4"] -> w381
          tunnel: [w411] -> w379
          tunnel: [w391] -> w378
          tunnel: [w388] -> w377
          tunnel: w375 -> [w410]
          tunnel: w374 -> [w408]
          tunnel: w373 -> [w406]
          tunnel: [w405] -> w372
          tunnel: w371 -> [w403]
          tunnel: [w402] -> w370
          tunnel: [w401] -> w369
          tunnel: [w400] -> w368
          tunnel: w366 -> [w396]
          tunnel: [w395] -> w365
          tunnel: [w393] -> w364
          tunnel: w381 -> [w427]
          tunnel: w380 -> [w425]
          tunnel: w379 -> [w424]
          tunnel: w378 -> [w423]
          tunnel: w377 -> [w422]
          tunnel: w376 -> [w421]
          tunnel: w370 -> [w450]
          tunnel: w368 -> [w449]
          tunnel: w367 -> [w448]
          frame #0 {
            n107 = Build Array (concatenate)(w396, "Temp 4") -> (w395:dbl[])
            n108 = Subtract(x=w410, y=1) -> (x-y=w394:i32)
            n109 = Index Array(array=w395, index=w394) -> (element=w393:dbl)
            n110 = Multiply(x=w394, y=w408) -> (x*y=w407:dbl)
            n111 = Add(x="O2 mole Frac 4", y="CH4/He mole frac 4") -> (x+y=w398:dbl)
            n112 = Quotient & Remainder(x=w407, y=w406) -> (floor(x/y)=w405:dbl)  [unwired: 1 out]
            n113 = Multiply(x="Total Flow 4", y="O2 mole Frac 4") -> (x*y=w411:dbl)
            "O2 Flow 4" <- w411
            n114 = Multiply(x="Total Flow 4", y="CH4/He mole frac 4") -> (x*y=w388:dbl)
            "CH4/He Actual Flow 4" <- w388
            n115 = Subtract(x=1, y=w398) -> (x-y=w413:dbl)
            "N2 mole frac 4" <- w413
            n116 = Number To Decimal String(number=w405) -> (decimal integer string=w404:string)  [unwired: 1 in]
            n117 = Build Array (concatenate)(w412, w413) -> (w401:dbl[])
            n118 = Multiply(x=w413, y="Total Flow 4") -> (x*y=w391:dbl)
            "N2 Actual Flow 4" <- w391
            n119 = Divide(x=w391, y=0.7027) -> (x/y=w390:dbl)
            "N2 Set Flow 4" <- w390
            n120 = Concatenate Strings(w403, w404) -> (w402:string)
            n121 = Index Array(array=w401, index=w394) -> (element=w400:dbl)
            n122 = Divide(x=w388, y=1.4819) -> (x/y=w387:dbl)
            "CH4/He Set Flow 4" <- w387
            "Exp 4" <- TRUE
          }
          frame #1 {
            # "Cat Mass"
            # "MFC 1,2,3"
            # "T"
            # "file"
            n123 = call <vilib>:"New Session.vi"("Path to Python Module (.py File)"=path "C:/Users/Solomon/Documents/Enthought/ResultFileGeneratorV2.py") -> ("error out"=w446:errorcluster, "Session ID out"=w447:T4)  [unwired: 9 in]
            n124 = call <vilib>:"Pack.vi"("Argument"=w425, "error in (no error)"=w446, "Session ID"=w447) -> ("error out"=w444:errorcluster, "Python Object References Out"=w443:T5, "Session ID out"=w445:T4)  [unwired: 6 in]
            n125 = call <vilib>:"Pack.vi"("Argument"=w427, "error in (no error)"=w444, "Python Object References In"=w443, "Session ID"=w445) -> ("error out"=w438:errorcluster, "Python Object References Out"=w439:T5, "Session ID out"=w440:T4)  [unwired: 5 in]
            n126 = call <vilib>:"Pack.vi"("Argument"=w424, "error in (no error)"=w438, "Python Object References In"=w439, "Session ID"=w440) -> ("error out"=w435:errorcluster, "Python Object References Out"=w436:T5, "Session ID out"=w437:T4)  [unwired: 5 in]
            n127 = call <vilib>:"Pack.vi"("Argument"=w423, "error in (no error)"=w435, "Python Object References In"=w436, "Session ID"=w437) -> ("error out"=w432:errorcluster, "Python Object References Out"=w433:T5, "Session ID out"=w434:T4)  [unwired: 5 in]
            n128 = call <vilib>:"Pack.vi"("Argument"=w422, "error in (no error)"=w432, "Python Object References In"=w433, "Session ID"=w434) -> ("error out"=w418:errorcluster, "Python Object References Out"=w419:T5, "Session ID out"=w420:T4)  [unwired: 5 in]
            n129 = call <vilib>:"Pack.vi"("Argument"=w421, "error in (no error)"=w418, "Python Object References In"=w419, "Session ID"=w420) -> ("error out"=w429:errorcluster, "Python Object References Out"=w430:T5, "Session ID out"=w431:T4)  [unwired: 5 in]
            n130 = call <vilib>:"Call.vi"("Function or Method Name"="AppendResultFile" ("Function Name"), "error in (no error)"=w429, "Python Object References In"=w430, "Session ID"=w431) -> ("error out"=w441:errorcluster, "Session ID out"=w442:T4)  [unwired: 5 in, 1 out]
            n131 = call <vilib>:"Close Session.vi"("error in (no error)"=w441, "Session ID"=w442) -> ()  [unwired: 9 in, 1 out]
          }
          frame #2 {
            n132 = call <vilib>:"New Session.vi"("Path to Python Module (.py File)"=path "C:/Users/Solomon/Documents/Methane_GC_forCSV.py") -> ("error out"=w461:errorcluster, "Session ID out"=w459:T4)  [unwired: 9 in]
            n133 = call <vilib>:"Pack.vi"("Argument"=w450, "error in (no error)"=w461, "Session ID"=w459) -> ("error out"=w464:errorcluster, "Python Object References Out"=w474:T5, "Session ID out"=w463:T4)  [unwired: 6 in]
            n134 = call <vilib>:"Pack.vi"("Argument"=w449, "error in (no error)"=w464, "Python Object References In"=w474, "Session ID"=w463) -> ("error out"=w455:errorcluster, "Python Object References Out"=w456:T5, "Session ID out"=w457:T4)  [unwired: 5 in]
            n135 = call <vilib>:"Pack.vi"("Argument"=w448, "error in (no error)"=w455, "Python Object References In"=w456, "Session ID"=w457) -> ("error out"=w454:errorcluster, "Python Object References Out"=w453:T5, "Session ID out"=w452:T4)  [unwired: 5 in]
            n136 = call <vilib>:"Call.vi"("Function or Method Name"="GC" ("Function Name"), "error in (no error)"=w454, "Python Object References In"=w453, "Session ID"=w452) -> ("error out"=w468:errorcluster, "Python Object References Out"=w475:T5, "Session ID out"=w465:T4)  [unwired: 5 in]
            n137 = call-poly <vilib>:"Unpack.vi"("error in (no error)"=w468, "Python Object References In"=w475, "Session ID"=w465) -> ("error out"=w469:errorcluster, "Value"=→"Measured CO2 mol fraction 3":dbl, "Python Object References Out"=w476:T5, "Session ID out"=w466:T4)  [unwired: 5 in]
            n138 = call-poly <vilib>:"Unpack.vi"("error in (no error)"=w469, "Python Object References In"=w476, "Session ID"=w466) -> ("error out"=w470:errorcluster, "Value"=→"Measured O2 mol fraction 3":dbl, "Python Object References Out"=w477:T5, "Session ID out"=w467:T4)  [unwired: 5 in]
            n139 = call-poly <vilib>:"Unpack.vi"("error in (no error)"=w470, "Python Object References In"=w477, "Session ID"=w467) -> ("error out"=w462:errorcluster, "Value"=→"Measured CH4 mol fraction 3":dbl, "Session ID out"=w460:T4)  [unwired: 5 in, 1 out]
            n140 = call <vilib>:"Close Session.vi"("error in (no error)"=w462, "Session ID"=w460) -> ()  [unwired: 9 in, 1 out]
          }
        }
      }
      frame 5 {
        n141 = flat-sequence {
          tunnel: ["Temp 5"] -> w500
          tunnel: w499 -> [w526]
          tunnel: [w525] -> w498
          tunnel: [w504] -> w497
          tunnel: [w501] -> w496
          tunnel: ["Temp 5"] -> w495
          tunnel: [w525] -> w493
          tunnel: [w505] -> w492
          tunnel: [w502] -> w491
          tunnel: w489 -> [w524]
          tunnel: w488 -> [w522]
          tunnel: w487 -> [w520]
          tunnel: [w519] -> w486
          tunnel: w485 -> [w517]
          tunnel: [w516] -> w484
          tunnel: [w515] -> w483
          tunnel: [w514] -> w482
          tunnel: w480 -> [w510]
          tunnel: [w509] -> w479
          tunnel: [w507] -> w478
          tunnel: w495 -> [w541]
          tunnel: w494 -> [w539]
          tunnel: w493 -> [w538]
          tunnel: w492 -> [w537]
          tunnel: w491 -> [w536]
          tunnel: w490 -> [w535]
          tunnel: w484 -> [w564]
          tunnel: w482 -> [w563]
          tunnel: w481 -> [w562]
          frame #0 {
            n142 = Build Array (concatenate)(w510, "Temp 5") -> (w509:dbl[])
            n143 = Subtract(x=w524, y=1) -> (x-y=w508:i32)
            n144 = Index Array(array=w509, index=w508) -> (element=w507:dbl)
            n145 = Multiply(x=w508, y=w522) -> (x*y=w521:dbl)
            n146 = Add(x="O2 mole Frac 5", y="CH4/He mole frac 5") -> (x+y=w512:dbl)
            n147 = Quotient & Remainder(x=w521, y=w520) -> (floor(x/y)=w519:dbl)  [unwired: 1 out]
            n148 = Multiply(x="Total Flow 5", y="O2 mole Frac 5") -> (x*y=w525:dbl)
            "O2 Flow 5" <- w525
            n149 = Multiply(x="Total Flow 5", y="CH4/He mole frac 5") -> (x*y=w502:dbl)
            "CH4/He Actual Flow 5" <- w502
            n150 = Subtract(x=1, y=w512) -> (x-y=w527:dbl)
            "N2 mole frac 5" <- w527
            n151 = Number To Decimal String(number=w519) -> (decimal integer string=w518:string)  [unwired: 1 in]
            n152 = Build Array (concatenate)(w526, w527) -> (w515:dbl[])
            n153 = Multiply(x=w527, y="Total Flow 5") -> (x*y=w505:dbl)
            "N2 Actual Flow 5" <- w505
            n154 = Concatenate Strings(w517, w518) -> (w516:string)
            n155 = Divide(x=w505, y=0.7027) -> (x/y=w504:dbl)
            "N2 Set Flow 5" <- w504
            n156 = Index Array(array=w515, index=w508) -> (element=w514:dbl)
            n157 = Divide(x=w502, y=1.4819) -> (x/y=w501:dbl)
            "CH4/He Set Flow 5" <- w501
            "Exp 5" <- TRUE
          }
          frame #1 {
            # "Cat Mass"
            # "MFC 1,2,3"
            # "T"
            # "file"
            n158 = call <vilib>:"New Session.vi"("Path to Python Module (.py File)"=path "C:/Users/Solomon/Documents/Enthought/ResultFileGeneratorV2.py") -> ("error out"=w560:errorcluster, "Session ID out"=w561:T4)  [unwired: 9 in]
            n159 = call <vilib>:"Pack.vi"("Argument"=w539, "error in (no error)"=w560, "Session ID"=w561) -> ("error out"=w558:errorcluster, "Python Object References Out"=w557:T5, "Session ID out"=w559:T4)  [unwired: 6 in]
            n160 = call <vilib>:"Pack.vi"("Argument"=w541, "error in (no error)"=w558, "Python Object References In"=w557, "Session ID"=w559) -> ("error out"=w552:errorcluster, "Python Object References Out"=w553:T5, "Session ID out"=w554:T4)  [unwired: 5 in]
            n161 = call <vilib>:"Pack.vi"("Argument"=w538, "error in (no error)"=w552, "Python Object References In"=w553, "Session ID"=w554) -> ("error out"=w549:errorcluster, "Python Object References Out"=w550:T5, "Session ID out"=w551:T4)  [unwired: 5 in]
            n162 = call <vilib>:"Pack.vi"("Argument"=w537, "error in (no error)"=w549, "Python Object References In"=w550, "Session ID"=w551) -> ("error out"=w546:errorcluster, "Python Object References Out"=w547:T5, "Session ID out"=w548:T4)  [unwired: 5 in]
            n163 = call <vilib>:"Pack.vi"("Argument"=w536, "error in (no error)"=w546, "Python Object References In"=w547, "Session ID"=w548) -> ("error out"=w532:errorcluster, "Python Object References Out"=w533:T5, "Session ID out"=w534:T4)  [unwired: 5 in]
            n164 = call <vilib>:"Pack.vi"("Argument"=w535, "error in (no error)"=w532, "Python Object References In"=w533, "Session ID"=w534) -> ("error out"=w543:errorcluster, "Python Object References Out"=w544:T5, "Session ID out"=w545:T4)  [unwired: 5 in]
            n165 = call <vilib>:"Call.vi"("Function or Method Name"="AppendResultFile" ("Function Name"), "error in (no error)"=w543, "Python Object References In"=w544, "Session ID"=w545) -> ("error out"=w555:errorcluster, "Session ID out"=w556:T4)  [unwired: 5 in, 1 out]
            n166 = call <vilib>:"Close Session.vi"("error in (no error)"=w555, "Session ID"=w556) -> ()  [unwired: 9 in, 1 out]
          }
          frame #2 {
            n167 = call <vilib>:"New Session.vi"("Path to Python Module (.py File)"=path "C:/Users/Solomon/Documents/Methane_GC_forCSV.py") -> ("error out"=w575:errorcluster, "Session ID out"=w573:T4)  [unwired: 9 in]
            n168 = call <vilib>:"Pack.vi"("Argument"=w564, "error in (no error)"=w575, "Session ID"=w573) -> ("error out"=w578:errorcluster, "Python Object References Out"=w588:T5, "Session ID out"=w577:T4)  [unwired: 6 in]
            n169 = call <vilib>:"Pack.vi"("Argument"=w563, "error in (no error)"=w578, "Python Object References In"=w588, "Session ID"=w577) -> ("error out"=w569:errorcluster, "Python Object References Out"=w570:T5, "Session ID out"=w571:T4)  [unwired: 5 in]
            n170 = call <vilib>:"Pack.vi"("Argument"=w562, "error in (no error)"=w569, "Python Object References In"=w570, "Session ID"=w571) -> ("error out"=w568:errorcluster, "Python Object References Out"=w567:T5, "Session ID out"=w566:T4)  [unwired: 5 in]
            n171 = call <vilib>:"Call.vi"("Function or Method Name"="GC" ("Function Name"), "error in (no error)"=w568, "Python Object References In"=w567, "Session ID"=w566) -> ("error out"=w582:errorcluster, "Python Object References Out"=w589:T5, "Session ID out"=w579:T4)  [unwired: 5 in]
            n172 = call-poly <vilib>:"Unpack.vi"("error in (no error)"=w582, "Python Object References In"=w589, "Session ID"=w579) -> ("error out"=w583:errorcluster, "Value"=→"Measured CO2 mol fraction 4":dbl, "Python Object References Out"=w590:T5, "Session ID out"=w580:T4)  [unwired: 5 in]
            n173 = call-poly <vilib>:"Unpack.vi"("error in (no error)"=w583, "Python Object References In"=w590, "Session ID"=w580) -> ("error out"=w584:errorcluster, "Value"=→"Measured O2 mol fraction 4":dbl, "Python Object References Out"=w591:T5, "Session ID out"=w581:T4)  [unwired: 5 in]
            n174 = call-poly <vilib>:"Unpack.vi"("error in (no error)"=w584, "Python Object References In"=w591, "Session ID"=w581) -> ("error out"=w576:errorcluster, "Value"=→"Measured CH4 mol fraction 4":dbl, "Session ID out"=w574:T4)  [unwired: 5 in, 1 out]
            n175 = call <vilib>:"Close Session.vi"("error in (no error)"=w576, "Session ID"=w574) -> ()  [unwired: 9 in, 1 out]
          }
        }
      }
      frame 6 {
        n176 = flat-sequence {
          tunnel: ["Temp 6"] -> w614
          tunnel: w613 -> [w640]
          tunnel: [w639] -> w612
          tunnel: [w618] -> w611
          tunnel: [w615] -> w610
          tunnel: ["Temp 6"] -> w609
          tunnel: [w639] -> w607
          tunnel: [w619] -> w606
          tunnel: [w616] -> w605
          tunnel: w603 -> [w638]
          tunnel: w602 -> [w636]
          tunnel: w601 -> [w634]
          tunnel: [w633] -> w600
          tunnel: w599 -> [w631]
          tunnel: [w630] -> w598
          tunnel: [w629] -> w597
          tunnel: [w628] -> w596
          tunnel: w594 -> [w624]
          tunnel: [w622] -> w593
          tunnel: [w621] -> w592
          tunnel: w609 -> [w655]
          tunnel: w608 -> [w653]
          tunnel: w607 -> [w652]
          tunnel: w606 -> [w651]
          tunnel: w605 -> [w650]
          tunnel: w604 -> [w649]
          tunnel: w598 -> [w678]
          tunnel: w596 -> [w677]
          tunnel: w595 -> [w676]
          frame #0 {
            n177 = Build Array (concatenate)(w624, "Temp 6") -> (w621:dbl[])
            n178 = Subtract(x=w638, y=1) -> (x-y=w623:i32)
            n179 = Index Array(array=w621, index=w623) -> (element=w622:dbl)
            n180 = Multiply(x=w623, y=w636) -> (x*y=w635:dbl)
            n181 = Add(x="O2 mole Frac 6", y="CH4/He mole frac 6") -> (x+y=w626:dbl)
            n182 = Quotient & Remainder(x=w635, y=w634) -> (floor(x/y)=w633:dbl)  [unwired: 1 out]
            n183 = Multiply(x="Total Flow 6", y="O2 mole Frac 6") -> (x*y=w639:dbl)
            "O2 Flow 6" <- w639
            n184 = Multiply(x="Total Flow 6", y="CH4/He mole frac 6") -> (x*y=w616:dbl)
            "CH4/He Actual Flow 6" <- w616
            n185 = Subtract(x=1, y=w626) -> (x-y=w641:dbl)
            "N2 mole frac 6" <- w641
            n186 = Number To Decimal String(number=w633) -> (decimal integer string=w632:string)  [unwired: 1 in]
            n187 = Build Array (concatenate)(w640, w641) -> (w629:dbl[])
            n188 = Multiply(x=w641, y="Total Flow 6") -> (x*y=w619:dbl)
            "N2 Actual Flow 6" <- w619
            n189 = Concatenate Strings(w631, w632) -> (w630:string)
            n190 = Divide(x=w619, y=0.7027) -> (x/y=w618:dbl)
            "N2 Set Flow 6" <- w618
            n191 = Divide(x=w616, y=1.4819) -> (x/y=w615:dbl)
            "CH4/He Set Flow 6" <- w615
            n192 = Index Array(array=w629, index=w623) -> (element=w628:dbl)
            "Exp 6" <- TRUE
          }
          frame #1 {
            # "Cat Mass"
            # "MFC 1,2,3"
            # "T"
            # "file"
            n193 = call <vilib>:"New Session.vi"("Path to Python Module (.py File)"=path "C:/Users/Solomon/Documents/Enthought/ResultFileGeneratorV2.py") -> ("error out"=w674:errorcluster, "Session ID out"=w675:T4)  [unwired: 9 in]
            n194 = call <vilib>:"Pack.vi"("Argument"=w653, "error in (no error)"=w674, "Session ID"=w675) -> ("error out"=w672:errorcluster, "Python Object References Out"=w671:T5, "Session ID out"=w673:T4)  [unwired: 6 in]
            n195 = call <vilib>:"Pack.vi"("Argument"=w655, "error in (no error)"=w672, "Python Object References In"=w671, "Session ID"=w673) -> ("error out"=w666:errorcluster, "Python Object References Out"=w667:T5, "Session ID out"=w668:T4)  [unwired: 5 in]
            n196 = call <vilib>:"Pack.vi"("Argument"=w652, "error in (no error)"=w666, "Python Object References In"=w667, "Session ID"=w668) -> ("error out"=w663:errorcluster, "Python Object References Out"=w664:T5, "Session ID out"=w665:T4)  [unwired: 5 in]
            n197 = call <vilib>:"Pack.vi"("Argument"=w651, "error in (no error)"=w663, "Python Object References In"=w664, "Session ID"=w665) -> ("error out"=w660:errorcluster, "Python Object References Out"=w661:T5, "Session ID out"=w662:T4)  [unwired: 5 in]
            n198 = call <vilib>:"Pack.vi"("Argument"=w650, "error in (no error)"=w660, "Python Object References In"=w661, "Session ID"=w662) -> ("error out"=w646:errorcluster, "Python Object References Out"=w647:T5, "Session ID out"=w648:T4)  [unwired: 5 in]
            n199 = call <vilib>:"Pack.vi"("Argument"=w649, "error in (no error)"=w646, "Python Object References In"=w647, "Session ID"=w648) -> ("error out"=w657:errorcluster, "Python Object References Out"=w658:T5, "Session ID out"=w659:T4)  [unwired: 5 in]
            n200 = call <vilib>:"Call.vi"("Function or Method Name"="AppendResultFile" ("Function Name"), "error in (no error)"=w657, "Python Object References In"=w658, "Session ID"=w659) -> ("error out"=w669:errorcluster, "Session ID out"=w670:T4)  [unwired: 5 in, 1 out]
            n201 = call <vilib>:"Close Session.vi"("error in (no error)"=w669, "Session ID"=w670) -> ()  [unwired: 9 in, 1 out]
          }
          frame #2 {
            n202 = call <vilib>:"New Session.vi"("Path to Python Module (.py File)"=path "C:/Users/Solomon/Documents/Methane_GC_forCSV.py") -> ("error out"=w689:errorcluster, "Session ID out"=w687:T4)  [unwired: 9 in]
            n203 = call <vilib>:"Pack.vi"("Argument"=w678, "error in (no error)"=w689, "Session ID"=w687) -> ("error out"=w692:errorcluster, "Python Object References Out"=w702:T5, "Session ID out"=w691:T4)  [unwired: 6 in]
            n204 = call <vilib>:"Pack.vi"("Argument"=w677, "error in (no error)"=w692, "Python Object References In"=w702, "Session ID"=w691) -> ("error out"=w683:errorcluster, "Python Object References Out"=w684:T5, "Session ID out"=w685:T4)  [unwired: 5 in]
            n205 = call <vilib>:"Pack.vi"("Argument"=w676, "error in (no error)"=w683, "Python Object References In"=w684, "Session ID"=w685) -> ("error out"=w682:errorcluster, "Python Object References Out"=w681:T5, "Session ID out"=w680:T4)  [unwired: 5 in]
            n206 = call <vilib>:"Call.vi"("Function or Method Name"="GC" ("Function Name"), "error in (no error)"=w682, "Python Object References In"=w681, "Session ID"=w680) -> ("error out"=w696:errorcluster, "Python Object References Out"=w703:T5, "Session ID out"=w693:T4)  [unwired: 5 in]
            n207 = call-poly <vilib>:"Unpack.vi"("error in (no error)"=w696, "Python Object References In"=w703, "Session ID"=w693) -> ("error out"=w697:errorcluster, "Value"=→"Measured CO2 mol fraction 5":dbl, "Python Object References Out"=w704:T5, "Session ID out"=w694:T4)  [unwired: 5 in]
            n208 = call-poly <vilib>:"Unpack.vi"("error in (no error)"=w697, "Python Object References In"=w704, "Session ID"=w694) -> ("error out"=w698:errorcluster, "Value"=→"Measured O2 mol fraction 5":dbl, "Python Object References Out"=w705:T5, "Session ID out"=w695:T4)  [unwired: 5 in]
            n209 = call-poly <vilib>:"Unpack.vi"("error in (no error)"=w698, "Python Object References In"=w705, "Session ID"=w695) -> ("error out"=w690:errorcluster, "Value"=→"Measured CH4 mol fraction 5":dbl, "Session ID out"=w688:T4)  [unwired: 5 in, 1 out]
            n210 = call <vilib>:"Close Session.vi"("error in (no error)"=w690, "Session ID"=w688) -> ()  [unwired: 9 in, 1 out]
          }
        }
      }
      frame 7 {
        n211 = flat-sequence {
          tunnel: ["Temp 7"] -> w728
          tunnel: w727 -> [w754]
          tunnel: [w753] -> w726
          tunnel: [w732] -> w725
          tunnel: [w729] -> w724
          tunnel: ["Temp 7"] -> w723
          tunnel: [w753] -> w721
          tunnel: [w733] -> w720
          tunnel: [w730] -> w719
          tunnel: w717 -> [w752]
          tunnel: w716 -> [w750]
          tunnel: w715 -> [w748]
          tunnel: [w747] -> w714
          tunnel: w713 -> [w745]
          tunnel: [w744] -> w712
          tunnel: [w743] -> w711
          tunnel: [w742] -> w710
          tunnel: w708 -> [w738]
          tunnel: [w737] -> w707
          tunnel: [w735] -> w706
          tunnel: w723 -> [w769]
          tunnel: w722 -> [w767]
          tunnel: w721 -> [w766]
          tunnel: w720 -> [w765]
          tunnel: w719 -> [w764]
          tunnel: w718 -> [w763]
          tunnel: w712 -> [w792]
          tunnel: w710 -> [w791]
          tunnel: w709 -> [w790]
          frame #0 {
            n212 = Build Array (concatenate)(w738, "Temp 7") -> (w737:dbl[])
            n213 = Subtract(x=w752, y=1) -> (x-y=w736:i32)
            n214 = Index Array(array=w737, index=w736) -> (element=w735:dbl)
            n215 = Multiply(x=w736, y=w750) -> (x*y=w749:dbl)
            n216 = Add(x="O2 mole Frac 7", y="CH4/He mole frac 7") -> (x+y=w740:dbl)
            n217 = Quotient & Remainder(x=w749, y=w748) -> (floor(x/y)=w747:dbl)  [unwired: 1 out]
            n218 = Multiply(x="Total Flow 7", y="O2 mole Frac 7") -> (x*y=w753:dbl)
            "O2 Flow 7" <- w753
            n219 = Multiply(x="Total Flow 7", y="CH4/He mole frac 7") -> (x*y=w730:dbl)
            "CH4/He Actual Flow 7" <- w730
            n220 = Subtract(x=1, y=w740) -> (x-y=w755:dbl)
            "N2 mole frac 7" <- w755
            n221 = Number To Decimal String(number=w747) -> (decimal integer string=w746:string)  [unwired: 1 in]
            n222 = Build Array (concatenate)(w754, w755) -> (w743:dbl[])
            n223 = Multiply(x=w755, y="Total Flow 7") -> (x*y=w733:dbl)
            "N2 Actual Flow 7" <- w733
            n224 = Concatenate Strings(w745, w746) -> (w744:string)
            n225 = Divide(x=w730, y=1.4819) -> (x/y=w729:dbl)
            "CH4/He Set Flow 7" <- w729
            n226 = Index Array(array=w743, index=w736) -> (element=w742:dbl)
            n227 = Divide(x=w733, y=0.7027) -> (x/y=w732:dbl)
            "N2 Set Flow 7" <- w732
            "Exp 7" <- TRUE
          }
          frame #1 {
            # "Cat Mass"
            # "MFC 1,2,3"
            # "T"
            # "file"
            n228 = call <vilib>:"New Session.vi"("Path to Python Module (.py File)"=path "C:/Users/Solomon/Documents/Enthought/ResultFileGeneratorV2.py") -> ("error out"=w788:errorcluster, "Session ID out"=w789:T4)  [unwired: 9 in]
            n229 = call <vilib>:"Pack.vi"("Argument"=w767, "error in (no error)"=w788, "Session ID"=w789) -> ("error out"=w786:errorcluster, "Python Object References Out"=w785:T5, "Session ID out"=w787:T4)  [unwired: 6 in]
            n230 = call <vilib>:"Pack.vi"("Argument"=w769, "error in (no error)"=w786, "Python Object References In"=w785, "Session ID"=w787) -> ("error out"=w780:errorcluster, "Python Object References Out"=w781:T5, "Session ID out"=w782:T4)  [unwired: 5 in]
            n231 = call <vilib>:"Pack.vi"("Argument"=w766, "error in (no error)"=w780, "Python Object References In"=w781, "Session ID"=w782) -> ("error out"=w777:errorcluster, "Python Object References Out"=w778:T5, "Session ID out"=w779:T4)  [unwired: 5 in]
            n232 = call <vilib>:"Pack.vi"("Argument"=w765, "error in (no error)"=w777, "Python Object References In"=w778, "Session ID"=w779) -> ("error out"=w774:errorcluster, "Python Object References Out"=w775:T5, "Session ID out"=w776:T4)  [unwired: 5 in]
            n233 = call <vilib>:"Pack.vi"("Argument"=w764, "error in (no error)"=w774, "Python Object References In"=w775, "Session ID"=w776) -> ("error out"=w760:errorcluster, "Python Object References Out"=w761:T5, "Session ID out"=w762:T4)  [unwired: 5 in]
            n234 = call <vilib>:"Pack.vi"("Argument"=w763, "error in (no error)"=w760, "Python Object References In"=w761, "Session ID"=w762) -> ("error out"=w771:errorcluster, "Python Object References Out"=w772:T5, "Session ID out"=w773:T4)  [unwired: 5 in]
            n235 = call <vilib>:"Call.vi"("Function or Method Name"="AppendResultFile" ("Function Name"), "error in (no error)"=w771, "Python Object References In"=w772, "Session ID"=w773) -> ("error out"=w783:errorcluster, "Session ID out"=w784:T4)  [unwired: 5 in, 1 out]
            n236 = call <vilib>:"Close Session.vi"("error in (no error)"=w783, "Session ID"=w784) -> ()  [unwired: 9 in, 1 out]
          }
          frame #2 {
            n237 = call <vilib>:"New Session.vi"("Path to Python Module (.py File)"=path "C:/Users/Solomon/Documents/Methane_GC_forCSV.py") -> ("error out"=w803:errorcluster, "Session ID out"=w801:T4)  [unwired: 9 in]
            n238 = call <vilib>:"Pack.vi"("Argument"=w792, "error in (no error)"=w803, "Session ID"=w801) -> ("error out"=w806:errorcluster, "Python Object References Out"=w816:T5, "Session ID out"=w805:T4)  [unwired: 6 in]
            n239 = call <vilib>:"Pack.vi"("Argument"=w791, "error in (no error)"=w806, "Python Object References In"=w816, "Session ID"=w805) -> ("error out"=w797:errorcluster, "Python Object References Out"=w798:T5, "Session ID out"=w799:T4)  [unwired: 5 in]
            n240 = call <vilib>:"Pack.vi"("Argument"=w790, "error in (no error)"=w797, "Python Object References In"=w798, "Session ID"=w799) -> ("error out"=w796:errorcluster, "Python Object References Out"=w795:T5, "Session ID out"=w794:T4)  [unwired: 5 in]
            n241 = call <vilib>:"Call.vi"("Function or Method Name"="GC" ("Function Name"), "error in (no error)"=w796, "Python Object References In"=w795, "Session ID"=w794) -> ("error out"=w810:errorcluster, "Python Object References Out"=w817:T5, "Session ID out"=w807:T4)  [unwired: 5 in]
            n242 = call-poly <vilib>:"Unpack.vi"("error in (no error)"=w810, "Python Object References In"=w817, "Session ID"=w807) -> ("error out"=w811:errorcluster, "Value"=→"Measured CO2 mol fraction 6":dbl, "Python Object References Out"=w818:T5, "Session ID out"=w808:T4)  [unwired: 5 in]
            n243 = call-poly <vilib>:"Unpack.vi"("error in (no error)"=w811, "Python Object References In"=w818, "Session ID"=w808) -> ("error out"=w812:errorcluster, "Value"=→"Measured O2 mol fraction 6":dbl, "Python Object References Out"=w819:T5, "Session ID out"=w809:T4)  [unwired: 5 in]
            n244 = call-poly <vilib>:"Unpack.vi"("error in (no error)"=w812, "Python Object References In"=w819, "Session ID"=w809) -> ("error out"=w804:errorcluster, "Value"=→"Measured CH4 mol fraction 6":dbl, "Session ID out"=w802:T4)  [unwired: 5 in, 1 out]
            n245 = call <vilib>:"Close Session.vi"("error in (no error)"=w804, "Session ID"=w802) -> ()  [unwired: 9 in, 1 out]
          }
        }
      }
      frame 8 {
        n246 = flat-sequence {
          tunnel: ["Temp 8"] -> w842
          tunnel: w841 -> [w868]
          tunnel: [w867] -> w840
          tunnel: [w846] -> w839
          tunnel: [w843] -> w838
          tunnel: ["Temp 8"] -> w837
          tunnel: [w867] -> w835
          tunnel: [w847] -> w834
          tunnel: [w844] -> w833
          tunnel: w831 -> [w866]
          tunnel: w830 -> [w864]
          tunnel: w829 -> [w862]
          tunnel: [w861] -> w828
          tunnel: w827 -> [w859]
          tunnel: [w858] -> w826
          tunnel: [w857] -> w825
          tunnel: [w856] -> w824
          tunnel: w822 -> [w852]
          tunnel: [w851] -> w821
          tunnel: [w849] -> w820
          tunnel: w837 -> [w883]
          tunnel: w836 -> [w881]
          tunnel: w835 -> [w880]
          tunnel: w834 -> [w879]
          tunnel: w833 -> [w878]
          tunnel: w832 -> [w877]
          tunnel: w826 -> [w906]
          tunnel: w824 -> [w905]
          tunnel: w823 -> [w904]
          frame #0 {
            n247 = Build Array (concatenate)(w852, "Temp 8") -> (w851:dbl[])
            n248 = Subtract(x=w866, y=1) -> (x-y=w850:i32)
            n249 = Index Array(array=w851, index=w850) -> (element=w849:dbl)
            n250 = Multiply(x=w850, y=w864) -> (x*y=w863:dbl)
            n251 = Add(x="O2 mole Frac 8", y="CH4/He mole frac 8") -> (x+y=w854:dbl)
            n252 = Quotient & Remainder(x=w863, y=w862) -> (floor(x/y)=w861:dbl)  [unwired: 1 out]
            n253 = Multiply(x="Total Flow 8", y="O2 mole Frac 8") -> (x*y=w867:dbl)
            "O2 Flow 8" <- w867
            n254 = Multiply(x="Total Flow 8", y="CH4/He mole frac 8") -> (x*y=w844:dbl)
            "CH4/He Actual Flow 8" <- w844
            n255 = Subtract(x=1, y=w854) -> (x-y=w869:dbl)
            "N2 mole frac 8" <- w869
            n256 = Number To Decimal String(number=w861) -> (decimal integer string=w860:string)  [unwired: 1 in]
            n257 = Build Array (concatenate)(w868, w869) -> (w857:dbl[])
            n258 = Multiply(x=w869, y="Total Flow 8") -> (x*y=w847:dbl)
            "N2 Actual Flow 8" <- w847
            n259 = Divide(x=w844, y=1.4819) -> (x/y=w843:dbl)
            "CH4/He Set Flow 8" <- w843
            n260 = Concatenate Strings(w859, w860) -> (w858:string)
            n261 = Index Array(array=w857, index=w850) -> (element=w856:dbl)
            n262 = Divide(x=w847, y=0.7027) -> (x/y=w846:dbl)
            "N2 Set Flow 8" <- w846
            "Exp 8" <- TRUE
          }
          frame #1 {
            # "Cat Mass"
            # "MFC 1,2,3"
            # "T"
            # "file"
            n263 = call <vilib>:"New Session.vi"("Path to Python Module (.py File)"=path "C:/Users/Solomon/Documents/Enthought/ResultFileGeneratorV2.py") -> ("error out"=w902:errorcluster, "Session ID out"=w903:T4)  [unwired: 9 in]
            n264 = call <vilib>:"Pack.vi"("Argument"=w881, "error in (no error)"=w902, "Session ID"=w903) -> ("error out"=w900:errorcluster, "Python Object References Out"=w899:T5, "Session ID out"=w901:T4)  [unwired: 6 in]
            n265 = call <vilib>:"Pack.vi"("Argument"=w883, "error in (no error)"=w900, "Python Object References In"=w899, "Session ID"=w901) -> ("error out"=w894:errorcluster, "Python Object References Out"=w895:T5, "Session ID out"=w896:T4)  [unwired: 5 in]
            n266 = call <vilib>:"Pack.vi"("Argument"=w880, "error in (no error)"=w894, "Python Object References In"=w895, "Session ID"=w896) -> ("error out"=w891:errorcluster, "Python Object References Out"=w892:T5, "Session ID out"=w893:T4)  [unwired: 5 in]
            n267 = call <vilib>:"Pack.vi"("Argument"=w879, "error in (no error)"=w891, "Python Object References In"=w892, "Session ID"=w893) -> ("error out"=w888:errorcluster, "Python Object References Out"=w889:T5, "Session ID out"=w890:T4)  [unwired: 5 in]
            n268 = call <vilib>:"Pack.vi"("Argument"=w878, "error in (no error)"=w888, "Python Object References In"=w889, "Session ID"=w890) -> ("error out"=w874:errorcluster, "Python Object References Out"=w875:T5, "Session ID out"=w876:T4)  [unwired: 5 in]
            n269 = call <vilib>:"Pack.vi"("Argument"=w877, "error in (no error)"=w874, "Python Object References In"=w875, "Session ID"=w876) -> ("error out"=w885:errorcluster, "Python Object References Out"=w886:T5, "Session ID out"=w887:T4)  [unwired: 5 in]
            n270 = call <vilib>:"Call.vi"("Function or Method Name"="AppendResultFile" ("Function Name"), "error in (no error)"=w885, "Python Object References In"=w886, "Session ID"=w887) -> ("error out"=w897:errorcluster, "Session ID out"=w898:T4)  [unwired: 5 in, 1 out]
            n271 = call <vilib>:"Close Session.vi"("error in (no error)"=w897, "Session ID"=w898) -> ()  [unwired: 9 in, 1 out]
          }
          frame #2 {
            n272 = call <vilib>:"New Session.vi"("Path to Python Module (.py File)"=path "C:/Users/Solomon/Documents/Methane_GC_forCSV.py") -> ("error out"=w917:errorcluster, "Session ID out"=w915:T4)  [unwired: 9 in]
            n273 = call <vilib>:"Pack.vi"("Argument"=w906, "error in (no error)"=w917, "Session ID"=w915) -> ("error out"=w920:errorcluster, "Python Object References Out"=w930:T5, "Session ID out"=w919:T4)  [unwired: 6 in]
            n274 = call <vilib>:"Pack.vi"("Argument"=w905, "error in (no error)"=w920, "Python Object References In"=w930, "Session ID"=w919) -> ("error out"=w911:errorcluster, "Python Object References Out"=w912:T5, "Session ID out"=w913:T4)  [unwired: 5 in]
            n275 = call <vilib>:"Pack.vi"("Argument"=w904, "error in (no error)"=w911, "Python Object References In"=w912, "Session ID"=w913) -> ("error out"=w910:errorcluster, "Python Object References Out"=w909:T5, "Session ID out"=w908:T4)  [unwired: 5 in]
            n276 = call <vilib>:"Call.vi"("Function or Method Name"="GC" ("Function Name"), "error in (no error)"=w910, "Python Object References In"=w909, "Session ID"=w908) -> ("error out"=w924:errorcluster, "Python Object References Out"=w931:T5, "Session ID out"=w921:T4)  [unwired: 5 in]
            n277 = call-poly <vilib>:"Unpack.vi"("error in (no error)"=w924, "Python Object References In"=w931, "Session ID"=w921) -> ("error out"=w925:errorcluster, "Value"=→"Measured CO2 mol fraction 7":dbl, "Python Object References Out"=w932:T5, "Session ID out"=w922:T4)  [unwired: 5 in]
            n278 = call-poly <vilib>:"Unpack.vi"("error in (no error)"=w925, "Python Object References In"=w932, "Session ID"=w922) -> ("error out"=w926:errorcluster, "Value"=→"Measured O2 mol fraction 7":dbl, "Python Object References Out"=w933:T5, "Session ID out"=w923:T4)  [unwired: 5 in]
            n279 = call-poly <vilib>:"Unpack.vi"("error in (no error)"=w926, "Python Object References In"=w933, "Session ID"=w923) -> ("error out"=w918:errorcluster, "Value"=→"Measured CH4 mol fraction 7":dbl, "Session ID out"=w916:T4)  [unwired: 5 in, 1 out]
            n280 = call <vilib>:"Close Session.vi"("error in (no error)"=w918, "Session ID"=w916) -> ()  [unwired: 9 in, 1 out]
          }
        }
      }
      frame 9 {
        n281 = flat-sequence {
          tunnel: [w967] -> w956
          tunnel: w955 -> [w983]
          tunnel: [w982] -> w954
          tunnel: [w960] -> w953
          tunnel: [w957] -> w952
          tunnel: [w967] -> w951
          tunnel: [w982] -> w949
          tunnel: [w961] -> w948
          tunnel: [w958] -> w947
          tunnel: w945 -> [w981]
          tunnel: w944 -> [w979]
          tunnel: w943 -> [w977]
          tunnel: [w976] -> w942
          tunnel: w941 -> [w974]
          tunnel: [w973] -> w940
          tunnel: [w972] -> w939
          tunnel: [w971] -> w938
          tunnel: w936 -> [w966]
          tunnel: [w965] -> w935
          tunnel: [w963] -> w934
          tunnel: w940 -> [w990]
          tunnel: w938 -> [w989]
          tunnel: w937 -> [w988]
          tunnel: w946 -> [_]
          tunnel: w947 -> [_]
          tunnel: w948 -> [_]
          tunnel: w949 -> [_]
          tunnel: w950 -> [_]
          tunnel: w951 -> [_]
          frame #0 {
            w968 = 0
            w967 = 0
            n282 = Build Array (concatenate)(w966, w967) -> (w965:dbl[])
            n283 = Subtract(x=w981, y=1) -> (x-y=w964:i32)
            n284 = Index Array(array=w965, index=w964) -> (element=w963:dbl)
            n285 = Multiply(x=w964, y=w979) -> (x*y=w978:dbl)
            n286 = Add(x="O2 mole Frac 9", y="CH4/He mole frac 9") -> (x+y=w969:dbl)
            n287 = Quotient & Remainder(x=w978, y=w977) -> (floor(x/y)=w976:dbl)  [unwired: 1 out]
            n288 = Multiply(x=w968, y="O2 mole Frac 9") -> (x*y=w982:dbl)
            "O2 Flow 9" <- w982
            n289 = Multiply(x=w968, y="CH4/He mole frac 9") -> (x*y=w958:dbl)
            "CH4/He Actual Flow 9" <- w958
            n290 = Subtract(x=1, y=w969) -> (x-y=w984:dbl)
            "N2 mole frac 9" <- w984
            n291 = Number To Decimal String(number=w976) -> (decimal integer string=w975:string)  [unwired: 1 in]
            n292 = Build Array (concatenate)(w983, w984) -> (w972:dbl[])
            n293 = Multiply(x=w984, y=w968) -> (x*y=w961:dbl)
            "N2 Actual Flow 9" <- w961
            n294 = Concatenate Strings(w974, w975) -> (w973:string)
            n295 = Index Array(array=w972, index=w964) -> (element=w971:dbl)
            n296 = Divide(x=w961, y=0.7027) -> (x/y=w960:dbl)
            "N2 Set Flow 9" <- w960
            n297 = Divide(x=w958, y=1.4819) -> (x/y=w957:dbl)
            "CH4/He Set Flow 9" <- w957
            "Exp 9" <- TRUE
          }
          frame #1 {
            n298 = call <vilib>:"New Session.vi"("Path to Python Module (.py File)"=path "C:/Users/Solomon/Documents/Methane_GC_forCSVLast.py") -> ("error out"=w1001:errorcluster, "Session ID out"=w999:T4)  [unwired: 9 in]
            n299 = call <vilib>:"Pack.vi"("Argument"=w990, "error in (no error)"=w1001, "Session ID"=w999) -> ("error out"=w1004:errorcluster, "Python Object References Out"=w1014:T5, "Session ID out"=w1003:T4)  [unwired: 6 in]
            n300 = call <vilib>:"Pack.vi"("Argument"=w989, "error in (no error)"=w1004, "Python Object References In"=w1014, "Session ID"=w1003) -> ("error out"=w995:errorcluster, "Python Object References Out"=w996:T5, "Session ID out"=w997:T4)  [unwired: 5 in]
            n301 = call <vilib>:"Pack.vi"("Argument"=w988, "error in (no error)"=w995, "Python Object References In"=w996, "Session ID"=w997) -> ("error out"=w994:errorcluster, "Python Object References Out"=w993:T5, "Session ID out"=w992:T4)  [unwired: 5 in]
            n302 = call <vilib>:"Call.vi"("Function or Method Name"="GCLast" ("Function Name"), "error in (no error)"=w994, "Python Object References In"=w993, "Session ID"=w992) -> ("error out"=w1008:errorcluster, "Python Object References Out"=w1015:T5, "Session ID out"=w1005:T4)  [unwired: 5 in]
            n303 = call-poly <vilib>:"Unpack.vi"("error in (no error)"=w1008, "Python Object References In"=w1015, "Session ID"=w1005) -> ("error out"=w1009:errorcluster, "Value"=→"Measured CO2 mol fraction 8":dbl, "Python Object References Out"=w1016:T5, "Session ID out"=w1006:T4)  [unwired: 5 in]
            n304 = call-poly <vilib>:"Unpack.vi"("error in (no error)"=w1009, "Python Object References In"=w1016, "Session ID"=w1006) -> ("error out"=w1010:errorcluster, "Value"=→"Measured O2 mol fraction 8":dbl, "Python Object References Out"=w1017:T5, "Session ID out"=w1007:T4)  [unwired: 5 in]
            n305 = call-poly <vilib>:"Unpack.vi"("error in (no error)"=w1010, "Python Object References In"=w1017, "Session ID"=w1007) -> ("error out"=w1002:errorcluster, "Value"=→"Measured CH4 mol fraction 8":dbl, "Session ID out"=w1000:T4)  [unwired: 5 in, 1 out]
            n306 = call <vilib>:"Close Session.vi"("error in (no error)"=w1002, "Session ID"=w1000) -> ()  [unwired: 9 in, 1 out]
          }
        }
      }
      frame 10, Default {
        n307 = flat-sequence {
          tunnel: [w1045] -> w1040
          tunnel: w1039 -> [w1063]
          tunnel: [w1062] -> w1038
          tunnel: [w1061] -> w1037
          tunnel: [w1060] -> w1036
          tunnel: [w1045] -> w1035
          tunnel: [w1062] -> w1033
          tunnel: [w1061] -> w1032
          tunnel: [w1060] -> w1031
          tunnel: w1029 -> [w1059]
          tunnel: w1028 -> [w1057]
          tunnel: w1027 -> [w1055]
          tunnel: [w1054] -> w1026
          tunnel: w1025 -> [w1052]
          tunnel: [w1051] -> w1024
          tunnel: [w1050] -> w1023
          tunnel: [w1049] -> w1022
          tunnel: w1020 -> [w1044]
          tunnel: [w1043] -> w1019
          tunnel: [w1041] -> w1018
          tunnel: w1024 -> [_]
          tunnel: w1022 -> [_]
          tunnel: w1021 -> [_]
          tunnel: w1030 -> [_]
          tunnel: w1031 -> [_]
          tunnel: w1032 -> [_]
          tunnel: w1033 -> [_]
          tunnel: w1034 -> [_]
          tunnel: w1035 -> [_]
          frame #0 {
            w1046 = 0
            w1045 = 0
            n308 = Build Array (concatenate)(w1044, w1045) -> (w1043:dbl[])
            n309 = Subtract(x=w1059, y=1) -> (x-y=w1042:i32)
            n310 = Index Array(array=w1043, index=w1042) -> (element=w1041:dbl)
            n311 = Multiply(x=w1042, y=w1057) -> (x*y=w1056:dbl)
            n312 = Add(x="O2 mole Frac 10", y="CH4/He mole frac 10") -> (x+y=w1047:dbl)
            n313 = Quotient & Remainder(x=w1056, y=w1055) -> (floor(x/y)=w1054:dbl)  [unwired: 1 out]
            n314 = Multiply(x=w1046, y="O2 mole Frac 10") -> (x*y=w1062:dbl)
            "O2 Flow 10" <- w1062
            n315 = Multiply(x=w1046, y="CH4/He mole frac 10") -> (x*y=w1060:dbl)
            "CH4/He Actual Flow 10" <- w1060
            n316 = Subtract(x=1, y=w1047) -> (x-y=w1064:dbl)
            "N2 mole frac 10" <- w1064
            n317 = Number To Decimal String(number=w1054) -> (decimal integer string=w1053:string)  [unwired: 1 in]
            n318 = Build Array (concatenate)(w1063, w1064) -> (w1050:dbl[])
            n319 = Multiply(x=w1064, y=w1046) -> (x*y=w1061:dbl)
            "N2 Actual Flow 10" <- w1061
            n320 = Concatenate Strings(w1052, w1053) -> (w1051:string)
            n321 = Index Array(array=w1050, index=w1042) -> (element=w1049:dbl)
            "Exp 10" <- TRUE
          }
          frame #1 {
          }
        }
      }
    }
    "Most recent GC number" <- w44
    "Previous temp" <- w33
    "New temp" <- w32
    n322 = node-c288(w62) -> (w67:T1)  [unwired: 3 in]
    n323 = timed-loop {
      tunnel: [w1147] -> w38
      tunnel: [w1146] -> w40
      tunnel: [w1103] -> w39
      tunnel: [w1133] -> w42
      tunnel: [w1132] -> w41
      timing: w67 -> [_]
      timing-out: [_] -> w66
      tunnel: w32 -> [w1116]
      tunnel: w65 -> [w1110]
      tunnel: w64 -> [w1109]
      tunnel: w63 -> [w1108]
      tunnel: w62 -> [w1106]
      tunnel: w61 -> [w1105]
      tunnel: w60 -> [w1104]
      tunnel: w59 -> [w1103]
      tunnel: w58 -> [w1102]
      tunnel: w55 -> [w1101]
      tunnel: w56 -> [w1100]
      tunnel: w57 -> [w1099]
      tunnel: "Exp Duration (min)" -> [w1097]
      tunnel: [w1083] -> w54
      tunnel: [w1083] -> w53
      tunnel: ["Shut Down Everything"] -> w51
      tunnel: "Result File Name (must include .xlsx)" -> [w1082]
      tunnel: w36 -> [w1073]
      tunnel: w33 -> [w1071]
      i -> [w1070]
      stop <- w1092 stop-if-true
      w1068 = 120
      w1089 = 3.0 ("y")
      w1090 = 430.0 ("y")
      w1120 = 3 ("Channel")
      w1121 = 2 ("Channel")
      w1122 = 1 ("Channel")
      w1123 = 5 ("COM")
      w1136 = 1.5685
      w1139 = 1.7476
      # "need to change it so it updates temperature all the time during the ramp stage"
      # "number of loops at half way point rounded to whole number"
      # "number of loops per exp"
      # "total exp time seconds"
      # "time per loop seconds"
      n324 = node-c288() -> ()  [unwired: 1 in, 1 out]
      n325 = Less?(x=w1070, y=w1068) -> (x < y?=w1072:bool)
      n326 = Divide(x=w1106, y=1000) -> (x/y=w1096:dbl)
      n327 = call-poly <vilib>:"DAQmx Read.vi"("task/channels in"=w1100, "error in"=w1099) -> ("task out"=w1133:refnum<k21>, "data"=w1141:dbl[], "error out"=w1132:errorcluster)  [unwired: 11 in]
      n328 = case shown="True" "Manual or Automatic" {
        tunnel: w1070 -> [_ w1174]
        tunnel: [FALSE w1172] -> w1112
        frame False {
        }
        frame True {
          n329 = Equal?(x=w1174, y=0) -> (x = y?=w1172:bool)
        }
      }
      n330 = Or(x="Update Flow set point", y=w1112) -> (x .or. y?=w1114:bool)
      n331 = Or(x=TRUE, y=w1112) -> (x .or. y?=w1115:bool)
      n332 = case shown="True" w1115 {
        tunnel: [w1196 w1207] -> w1145
        tunnel: [w1195 w1206] -> w1148
        tunnel: w1101 -> [w1195 w1205]
        tunnel: w1102 -> [w1196 w1204]
        tunnel: w1105 -> [_ w1203]
        tunnel: "Manual or Automatic" -> [_ w1202]
        tunnel: w1116 -> [_ w1201]
        tunnel: w1072 -> [_ w1200]
        tunnel: w1071 -> [_ w1199]
        tunnel: w1070 -> [_ w1198]
        tunnel: w1068 -> [_ w1197]
        frame False {
        }
        frame True {
          n333 = case shown="True" w1202 {
            tunnel: ["Target Temperaure value" w1213] -> w1208
            tunnel: w1201 -> [_ w1214]
            tunnel: w1200 -> [_ w1215]
            tunnel: w1199 -> [_ w1212]
            tunnel: w1198 -> [_ w1211]
            tunnel: w1197 -> [_ w1210]
            frame False {
            }
            frame True {
              n334 = case shown="False" w1215 {
                tunnel: w1214 -> [w1216 w1224]
                tunnel: [w1216 w1222] -> w1213
                tunnel: w1212 -> [_ w1223]
                tunnel: w1211 -> [_ w1220]
                tunnel: w1210 -> [_ w1217]
                frame False {
                }
                frame True {
                  n335 = Subtract(x=w1224, y=w1223) -> (x-y=w1219:dbl)
                  n336 = Divide(x=w1219, y=w1217) -> (x/y=w1218:dbl)
                  n337 = Multiply(x=w1218, y=w1220) -> (x*y=w1221:dbl)
                  n338 = Add(x=w1223, y=w1221) -> (x+y=w1222:dbl)
                }
              }
            }
          }
          n339 = call "CN7500_Write Set Point Value.vi"("Target Set Point Value"=w1208, "error in (no error)"=w1204, "Controller Number"=w1203, "VISA In"=w1205) -> ("error out"=w1207:errorcluster, "VISA Out"=w1206:refnum<visa-resource-name>)  [unwired: 6 in]
        }
      }
      n340 = case shown="True" w1114 {
        tunnel: w1123 -> [_ w1186]
        tunnel: w1122 -> [_ w1188]
        tunnel: w1121 -> [_ w1187]
        tunnel: w1120 -> [_ w1185]
        tunnel: "Manual or Automatic" -> [_ w1177]
        tunnel: w1110 -> [_ w1180]
        tunnel: w1109 -> [_ w1179]
        tunnel: w1108 -> [_ w1178]
        frame False {
        }
        frame True {
          w1184 = 2 ("DP")
          n341 = case shown="True" w1177 {
            tunnel: ["SetPoint Ch 1" w1194] -> w1181
            tunnel: ["SetPoint Ch2" w1193] -> w1182
            tunnel: ["SetPoint Ch3" w1192] -> w1183
            tunnel: w1180 -> [_ w1194]
            tunnel: w1179 -> [_ w1193]
            tunnel: w1178 -> [_ w1192]
            frame False {
            }
            frame True {
            }
          }
          n342 = dll-call lib="C:/Program Files/National Instruments/LabVIEW 2018/instr.lib/Brooks DLL 64bit/0254 64bit/BrooksDLL64.dll" fn="WriteSetPoint_0254"("COM"=w1186, "Channel"=w1188, "DP"=w1184, "SetPoint"=w1181) -> ()  [unwired: 8 in, 2 out]
          n343 = dll-call lib="C:/Program Files/National Instruments/LabVIEW 2018/instr.lib/Brooks DLL 64bit/0254 64bit/BrooksDLL64.dll" fn="WriteSetPoint_0254"("COM"=w1186, "Channel"=w1185, "DP"=w1184, "SetPoint"=w1183) -> ()  [unwired: 8 in, 2 out]
          n344 = dll-call lib="C:/Program Files/National Instruments/LabVIEW 2018/instr.lib/Brooks DLL 64bit/0254 64bit/BrooksDLL64.dll" fn="WriteSetPoint_0254"("COM"=w1186, "Channel"=w1187, "DP"=w1184, "SetPoint"=w1182) -> ()  [unwired: 8 in, 2 out]
        }
      }
      n345 = Index Array(array=w1141, index=0) -> (element=w1140:dbl)
      n346 = Index Array(array=w1141, index=1) -> (element=w1138:dbl)
      n347 = Multiply(x=w1140, y=w1139) -> (x*y=w1137:dbl)
      n348 = Multiply(x=w1139, y=w1138) -> (x*y=w1135:dbl)
      n349 = Add(x=w1136, y=w1135) -> (x+y=w1080:dbl)
      "Outlet Pressure (Bar g) 2" <- w1080
      n350 = Add(x=w1137, y=w1136) -> (x+y=w1081:dbl)
      "Inlet Pressure (Bar g) 3" <- w1081
      n351 = Merge Signals(w1081, w1080) -> (→"Pressure":dynamicdata)
      n352 = Multiply(x=w1097, y=60) -> (x*y=w1095:dbl)
      n353 = call "CN7500_Read Process Value.vi"("error in (no error)"=w1145, "Controller Number"=w1104, "VISA In"=w1148) -> ("error out"=w1146:errorcluster, "Set Point Value"=w1131:dbl, "Process Value"=w1091:dbl, "VISA Out"=w1147:refnum<visa-resource-name>)  [unwired: 5 in]
      "Temp Process Value" <- w1091
      n354 = Divide(x=w1095, y=w1096) -> (x/y=w1079:dbl)
      n355 = Merge Signals(w1091, w1131) -> (→"Temperature":dynamicdata)
      n356 = Greater?(x=w1070, y=w1079) -> (0:w1094:bool)
      n357 = dll-call lib="C:/Program Files/National Instruments/LabVIEW 2018/instr.lib/Brooks DLL 64bit/0254 64bit/BrooksDLL64.dll" fn="ReadSetPoint_0254"("COM"=w1123, "Channel"=w1122) -> ("Channel"=w1129:i32, "SetPoint"=→"Read SetPoint Ch1":sgl)  [unwired: 6 in, 2 out]
      n358 = dll-call lib="C:/Program Files/National Instruments/LabVIEW 2018/instr.lib/Brooks DLL 64bit/0254 64bit/BrooksDLL64.dll" fn="ReadSetPoint_0254"("COM"=w1123, "Channel"=w1121) -> ("Channel"=w1126:i32, "SetPoint"=→"Read SetPoint Ch2":sgl)  [unwired: 6 in, 2 out]
      n359 = dll-call lib="C:/Program Files/National Instruments/LabVIEW 2018/instr.lib/Brooks DLL 64bit/0254 64bit/BrooksDLL64.dll" fn="ReadSetPoint_0254"("COM"=w1123, "Channel"=w1120) -> ("Channel"=w1124:i32, "SetPoint"=→"Read SetPoint Ch3":sgl)  [unwired: 6 in, 2 out]
      n360 = Quotient & Remainder(x=w1079, y=2) -> (floor(x/y)=w1077:dbl)  [unwired: 1 out]
      n361 = Or(x="Shut Down Everything", y=w1094) -> (x .or. y?=w1088:bool)
      n362 = dll-call lib="C:/Program Files/National Instruments/LabVIEW 2018/instr.lib/Brooks DLL 64bit/0254 64bit/BrooksDLL64.dll" fn="ReadProcessVariable_0254"("COM"=w1123, "Channel"=w1129) -> ("PV"=w1119:sgl)  [unwired: 7 in, 2 out]
      "Process Value Ch1" <- w1119
      n363 = Or(x=w1088, y="Skip Experiment") -> (x .or. y?=w1086:bool)
      n364 = dll-call lib="C:/Program Files/National Instruments/LabVIEW 2018/instr.lib/Brooks DLL 64bit/0254 64bit/BrooksDLL64.dll" fn="ReadProcessVariable_0254"("COM"=w1123, "Channel"=w1126) -> ("PV"=w1118:sgl)  [unwired: 7 in, 2 out]
      "Process Value Ch2" <- w1118
      n365 = Equal?(x=w1070, y=w1077) -> (x = y?=w1076:bool)
      n366 = dll-call lib="C:/Program Files/National Instruments/LabVIEW 2018/instr.lib/Brooks DLL 64bit/0254 64bit/BrooksDLL64.dll" fn="ReadProcessVariable_0254"("COM"=w1123, "Channel"=w1124) -> ("PV"=w1117:sgl)  [unwired: 7 in, 2 out]
      "Process Value Ch3" <- w1117
      n367 = Merge Signals(w1091, w1131, w1081, w1080, w1119, w1118, w1117) -> (w1130:dynamicdata)
      n368 = call "Write To Measurement File"("Signals"=w1130) -> ()  [unwired: 16 in, 3 out]
      n369 = Greater?(x=w1081, y=w1089) -> (0:w1084:bool)
      "Pressure ShutDown Limit Reached" <- w1084
      n370 = Greater?(x=w1091, y=w1090) -> (0:w1083:bool)
      "Temp ShutDown Limit Reached" <- w1083
      n371 = Or(x=w1083, y=w1086) -> (x .or. y?=w1093:bool)
      n372 = Or(x=w1093, y=w1084) -> (x .or. y?=w1092:bool)
      n373 = Equal?(x=w1073, y=0.0) -> (x = y?=w1075:bool)
      n374 = case shown="False" w1075 {
        tunnel: w1082 -> [w1152 _]
        tunnel: w1081 -> [w1151 _]
        tunnel: w1080 -> [w1150 _]
        tunnel: w1076 -> [w1149 _]
        frame False {
          n375 = case shown="True" w1149 {
            tunnel: w1152 -> [_ w1156]
            tunnel: w1151 -> [_ w1155]
            tunnel: w1150 -> [_ w1154]
            frame False {
            }
            frame True {
              # "Pout"
              # "Pin"
              # "filename"
              n376 = call <vilib>:"New Session.vi"("Path to Python Module (.py File)"=path "C:/Users/Solomon/Documents/Enthought/PressureExcelWriter.py") -> ("error out"=w1168:errorcluster, "Session ID out"=w1169:T4)  [unwired: 9 in]
              n377 = call <vilib>:"Pack.vi"("Argument"=w1156, "error in (no error)"=w1168, "Session ID"=w1169) -> ("error out"=w1167:errorcluster, "Python Object References Out"=w1160:T5, "Session ID out"=w1164:T4)  [unwired: 6 in]
              n378 = call <vilib>:"Pack.vi"("Argument"=w1155, "error in (no error)"=w1167, "Python Object References In"=w1160, "Session ID"=w1164) -> ("error out"=w1166:errorcluster, "Python Object References Out"=w1159:T5, "Session ID out"=w1163:T4)  [unwired: 5 in]
              n379 = call <vilib>:"Pack.vi"("Argument"=w1154, "error in (no error)"=w1166, "Python Object References In"=w1159, "Session ID"=w1163) -> ("error out"=w1165:errorcluster, "Python Object References Out"=w1158:T5, "Session ID out"=w1162:T4)  [unwired: 5 in]
              n380 = call <vilib>:"Call.vi"("Function or Method Name"="AppendPressures" ("Function Name"), "error in (no error)"=w1165, "Python Object References In"=w1158, "Session ID"=w1162) -> ("error out"=w1170:errorcluster, "Session ID out"=w1161:T4)  [unwired: 5 in, 1 out]
              n381 = call <vilib>:"Close Session.vi"("error in (no error)"=w1170, "Session ID"=w1161) -> ()  [unwired: 9 in, 1 out]
            }
          }
        }
        frame True {
        }
      }
      n382 = node-c288() -> ()  [unwired: 1 in, 1 out]
      "Loop Count" <- w1070
      "Shut down Temperature" <- w1090
      "Pressure safety shut down" <- w1089
    }
    n383 = node-c288(w66) -> ()  [unwired: 1 out]
    n384 = Or(x=w54, y=w53) -> (x .or. y?=w52:bool)
    n385 = Or(x=w52, y=w51) -> (x .or. y?=w50:bool)
  }
  n386 = call <vilib>:"DAQmx Stop Task.vi"("task/channels in"=w8, "error in"=w7) -> ("task out"=w9:refnum<k21>, "error out"=w10:errorcluster)  [unwired: 12 in]
  n387 = call "CN7500_Write Set Point Value.vi"("Target Set Point Value"=0.0, "error in (no error)"=w3, "Controller Number"=w2, "VISA In"=w1) -> ("error out"=w6:errorcluster, "VISA Out"=w5:refnum<visa-resource-name>)  [unwired: 6 in]
  n388 = call "CN7500_Close.vi"("error in (no error)"=w6, "VISA resource name"=w5) -> ()  [unwired: 9 in, 1 out]
  n389 = call <vilib>:"DAQmx Clear Task.vi"("task in"=w9, "error in"=w10) -> ()  [unwired: 13 in, 1 out]
